vi "newGUI.vi"() -> ()   [LabVIEW 2021]
uses:
  UI Data.ctl
  Data.ctl
  <vilib>/Instr/_visa.llb/VISA Flush IO Buffer Mask.ctl
  f08f8e5a-3cc6-4510-ab96-cacb044e89f4.vi
  816ef2ce-0aac-4e16-9f0f-254035a33ee7.vi
  7bf0c881-b533-49c5-b976-3a179d9b9c35.vi
  5e66b44c-e304-46e7-babf-65c984714624.vi
  a6c2df6f-6ad4-4eb4-a9bc-2f05b466e969.vi
  d2f15d41-d429-4762-bc4d-8d0cbb89ed83.vi
  535851f3-05c5-415e-8a07-50860e4f08cf.vi
  3643a199-7bcb-4f24-a83d-5ca93d957abf.vi
  187f9bc3-0ed3-4701-b56c-3ff7ee860393.vi
  eb7b7dfd-645e-46e6-868f-ba0f7f713db4.vi
  <vilib>/Instr/_visa.llb/VISA Configure Serial Port (Instr).vi
  styles/colors.vi
  <vilib>/ULx/ULx_LV.dll
  <vilib>/ULx/Write.llb/ULx Write (Digital Bool 1Line 1Point).vi
  <vilib>/NI/Progress Bar/Progress Bar.lvlib
  <vilib>/zip/NI_Unzip.lvlib
  <vilib>/ULx/Create Channel.llb/ULx Create Channel (DO-Digital Output).vi
panel:
  in  "Stop button":bool
  in  "Run button":bool
  in  "Settings button":bool
  out "Console":string
  in  "Serial communication\n settings":T1={"COM"="", "baud rate"=115200, "data bits"=8, "parity"=enum."None", "stop bits"=10, "flow control"=enum."None", "delay"=50, "I/O channel"=""} {"stop bits" items=["1.0"=10, "1.5"=15, "2.0"=20]; "baud rate" max=921600; "data bits" max=16}
  in  "Paths":bool
  in  "Save button":bool
  in  "Path: 4.9.12.XXXX":path=path "C:/Users/ken_X/Documents/LabVIEW projects/Project-A/outset-medical/4.9.12.6034"
  in  "Path: Android OS":path=path "C:/Users/ken_X/Documents/LabVIEW projects/Project-A/outset-medical/Android OS"
  # "Serial communication\n settings"
  # "I/O Channel"
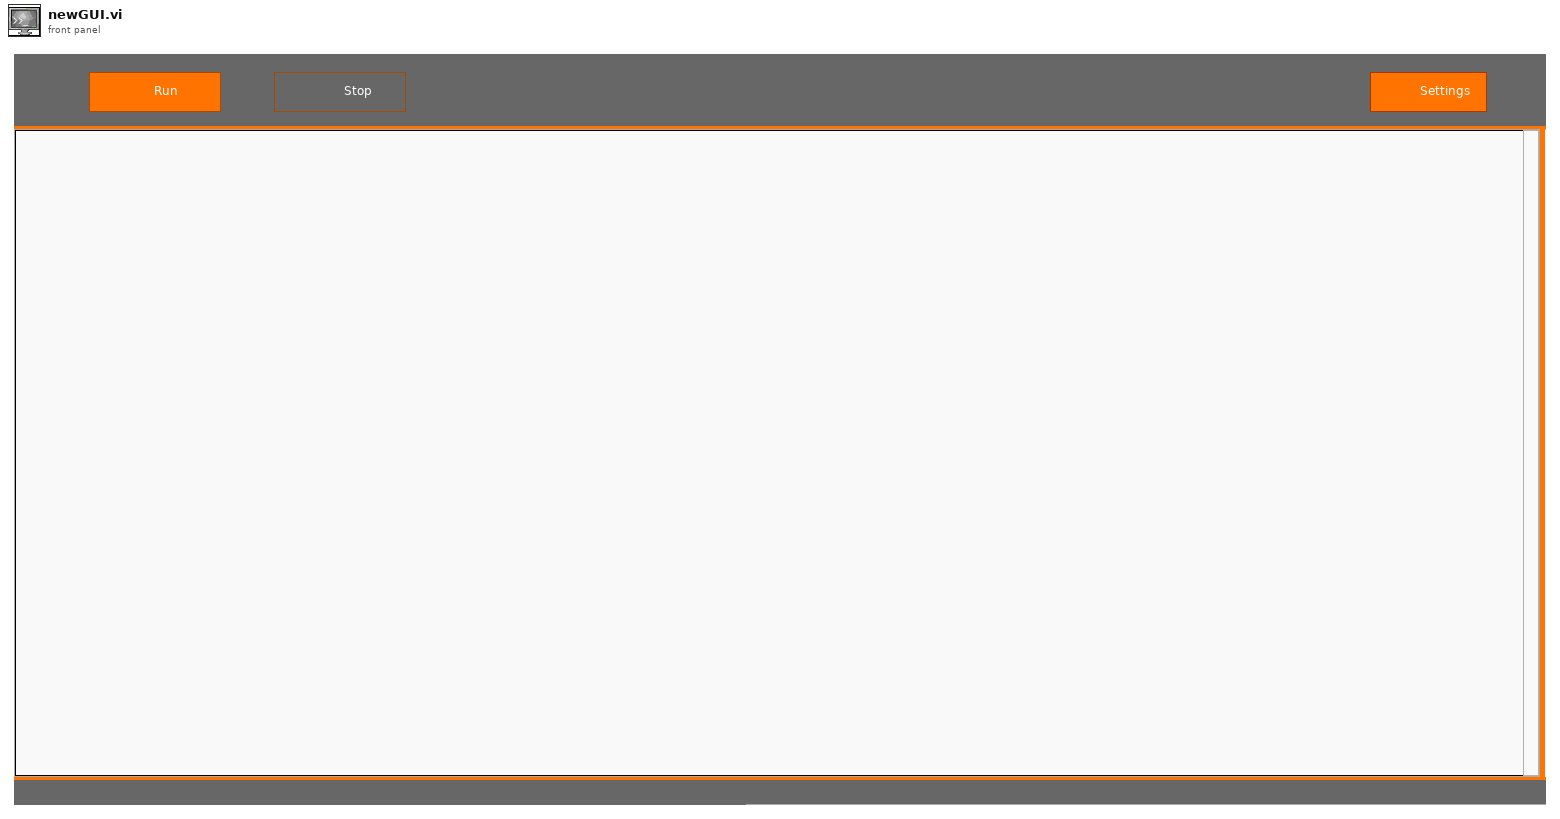
[diagram p1: front panel]
types:
  T1 = cluster{"COM":refnum<visa-resource-name>, "baud rate":u32, "data bits":u8, "parity":enum16{"None", "Odd", "Even", "Mark", "Space"}, "stop bits":u16, "flow control":enum16{"None", "XON/XOFF", "RTS/CTS", "DTR/DSR"}, "delay":u16, "I/O channel":refnum<k21>}
  T2 = typedef "Data.ctl" = cluster{"Console":refnum<vi>, "COM":refnum<visa-resource-name>, "Delay":u32, "IO task":refnum<k24>, "Python session":refnum<k35>, "Script path":path, "Media Url":string, "Media version":i32, "Attempts left":i32, "Version path":path, "Android path":path, "Python 2.7":path, "My temp":path}
  T3 = enum8{"Enabled", "Disabled", "Disabled and Grayed Out"}
  T4 = typedef "UI Data.ctl" = cluster{"settings splitter":refnum<vi>, "footer splitter":refnum<vi>, "Serial communication\n settings":refnum<vi>, "Path: Android OS":refnum<vi>, "Path: 4.9.12.XXXX":refnum<vi>}
  T5 = cluster{"primary color":u32, "secondary color":u32, "accent color":u32, "background color":u32, "accent s color":u32}
  T6 = cluster{"accent s color":u32, "accent s color":u32}
  T7 = cluster{"accent s color":u32, "accent color":u32}
  T8 = cluster{"primary color":u32, "primary color":u32}
  T9 = enum16{"open", "replace", "create", "open or create", "replace or create", "replace or create with confirmation"}
  T10 = cluster{"Android":path, "Version":path, "Labview Script":path, "Python 2.7":path, "My temp":path}
  T11 = typedef "VISA Flush IO Buffer Mask.ctl" = u16
  T12 = cluster{"secondary color":u32, "secondary color":u32}
  T13 = cluster{"Value":path, "Value":path, path, path, path}
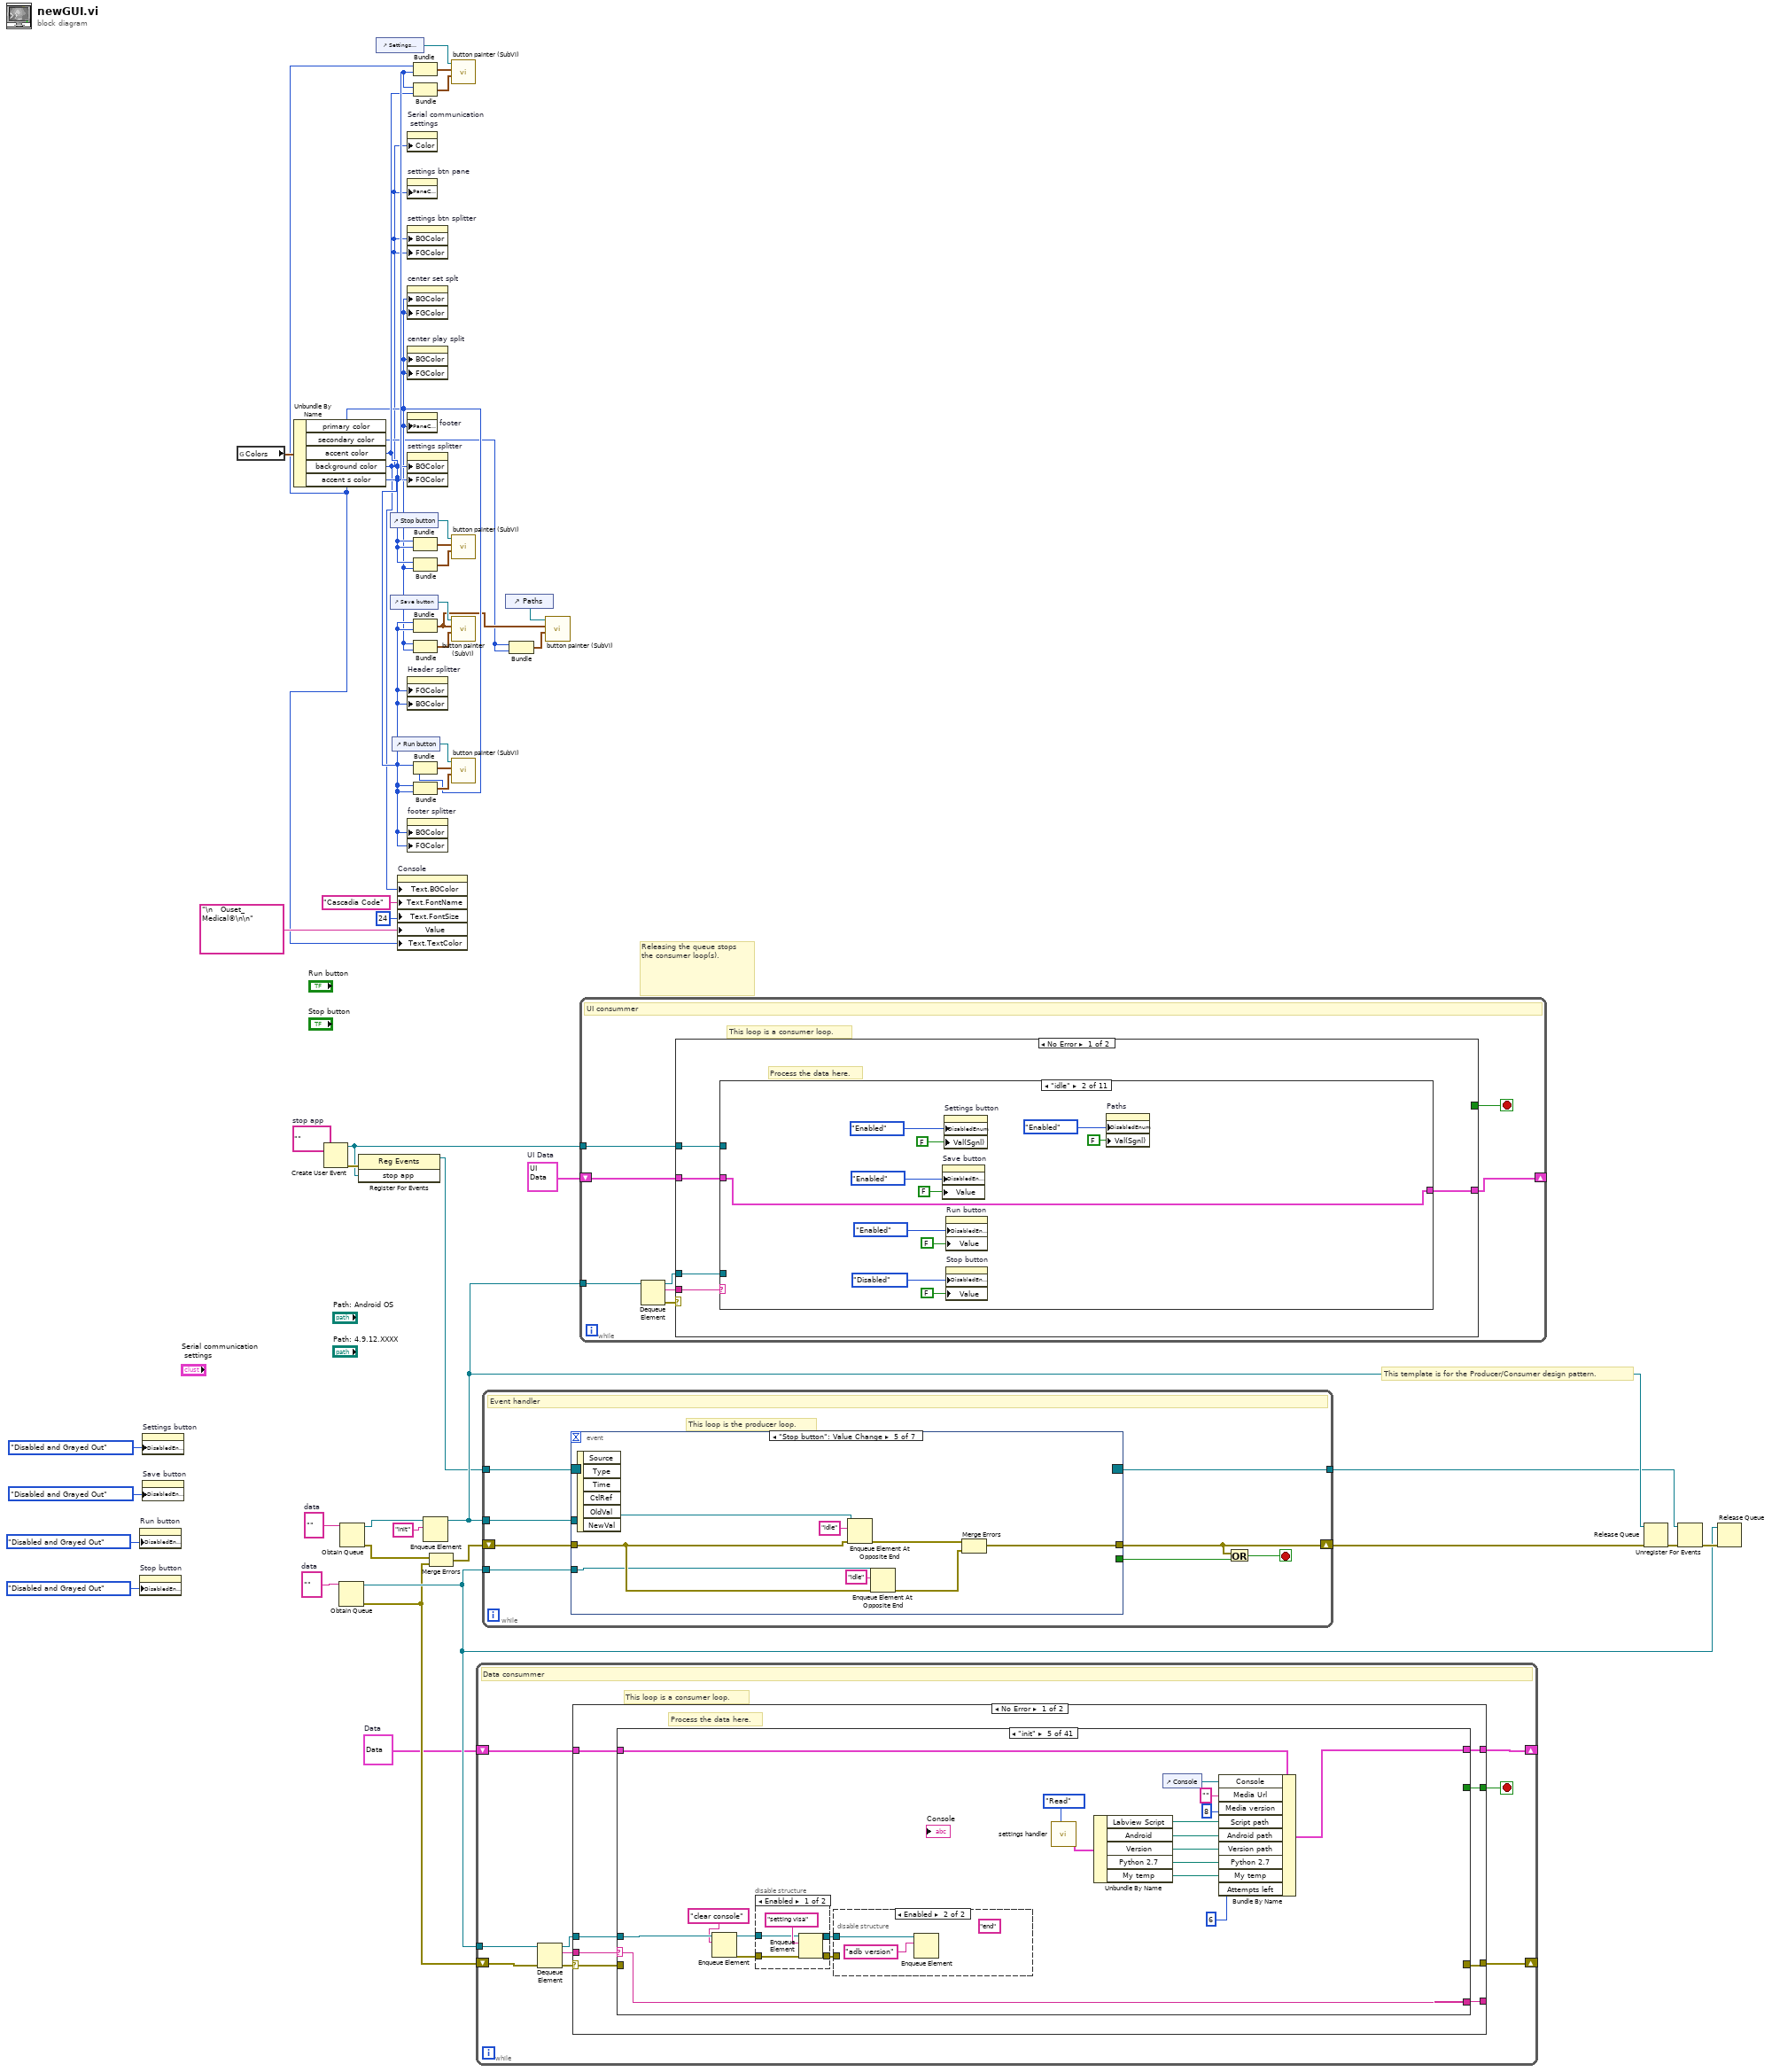
[diagram p0: block diagram]
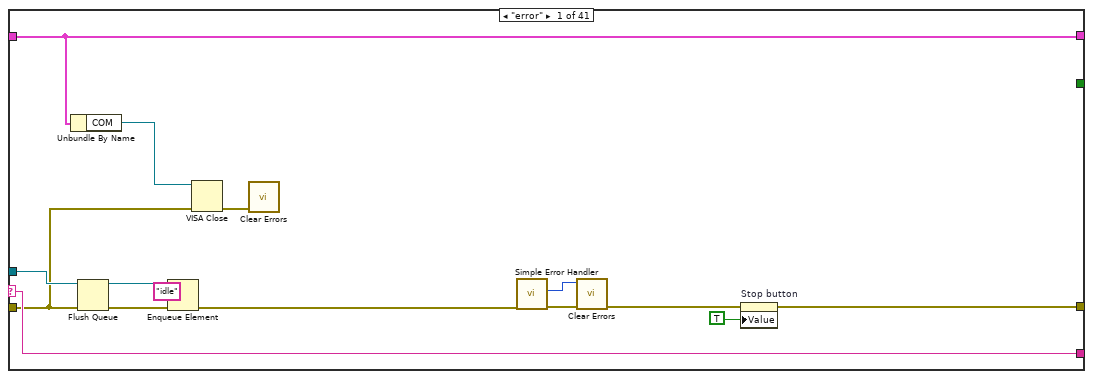
[diagram p2: hidden frame]
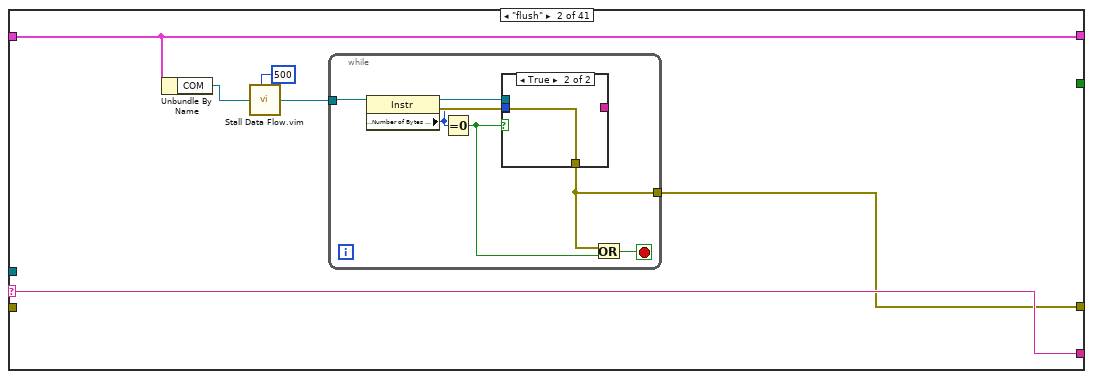
[diagram p3: hidden frame]
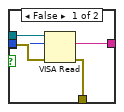
[diagram p4: hidden frame]
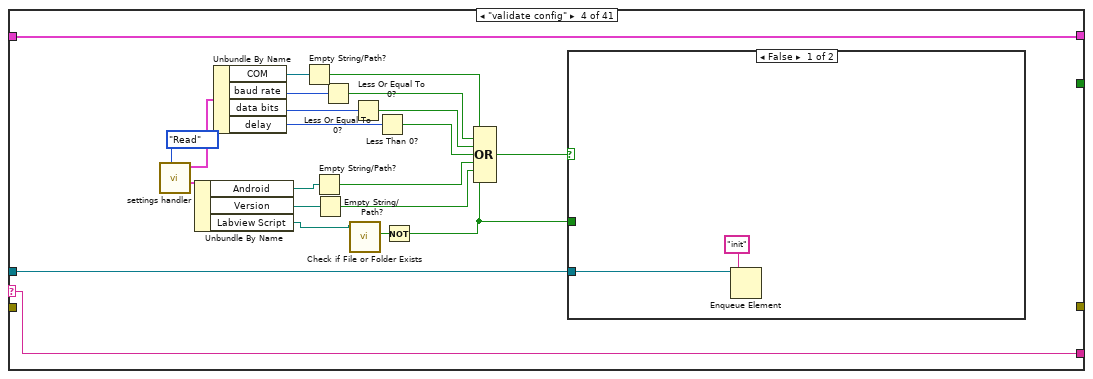
[diagram p6: hidden frame]
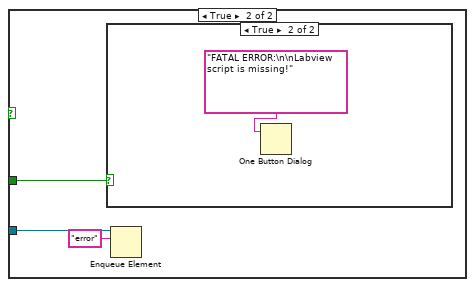
[diagram p7: hidden frame]
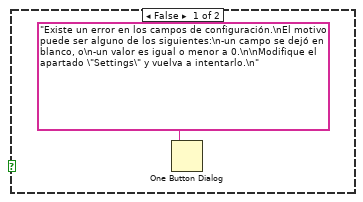
[diagram p8: hidden frame]
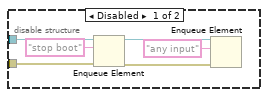
[diagram p10: hidden frame]
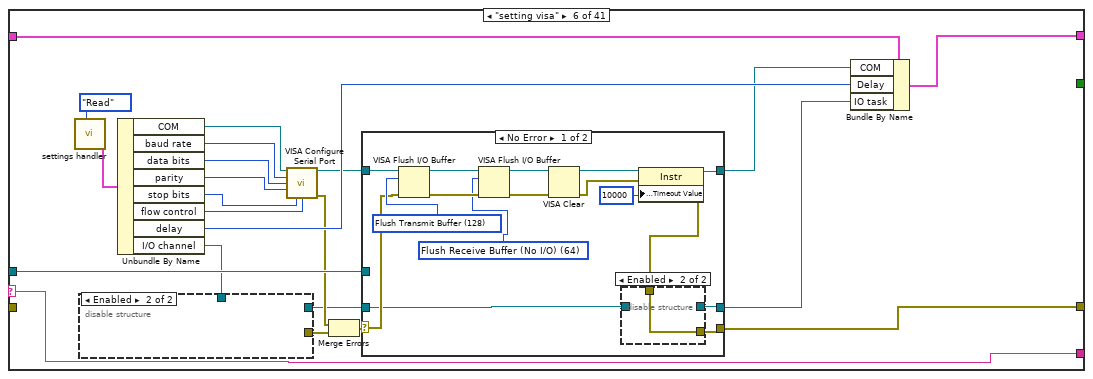
[diagram p11: hidden frame]
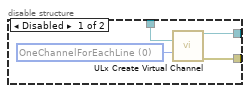
[diagram p12: hidden frame]
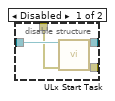
[diagram p13: hidden frame]
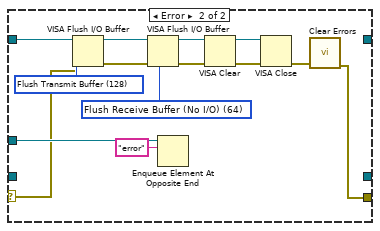
[diagram p14: hidden frame]
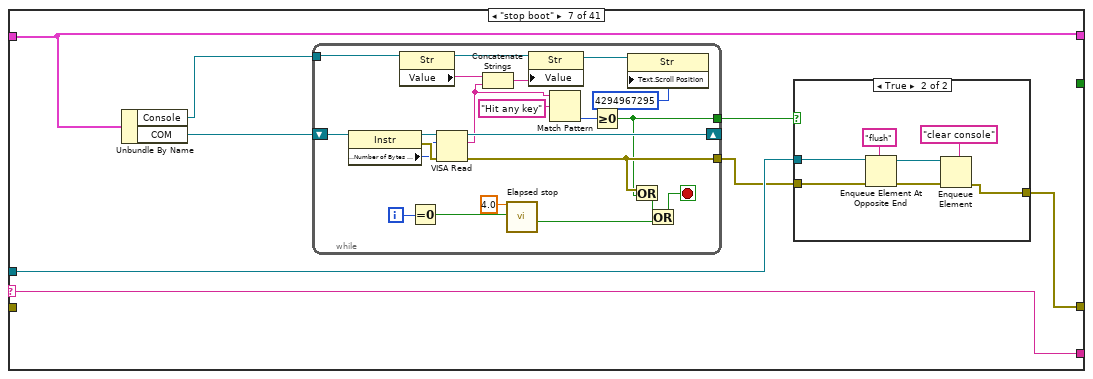
[diagram p15: hidden frame]
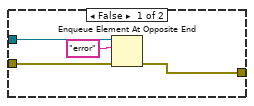
[diagram p16: hidden frame]
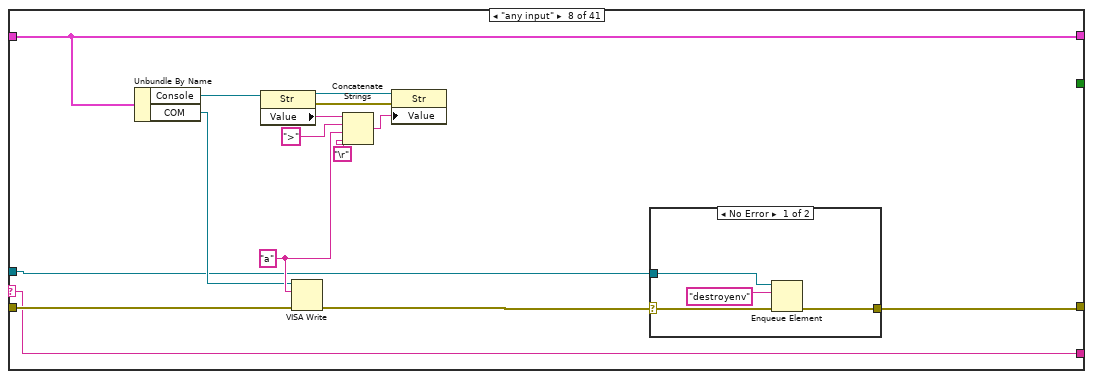
[diagram p17: hidden frame]
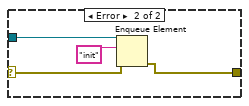
[diagram p18: hidden frame]
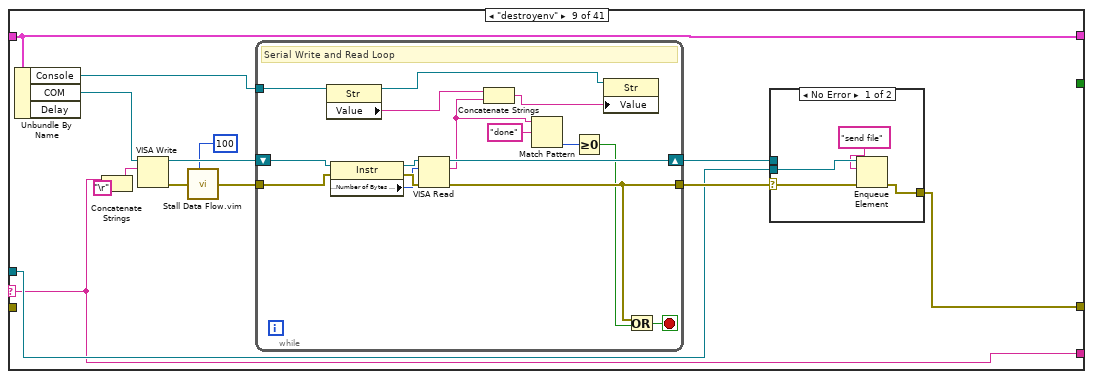
[diagram p19: hidden frame]
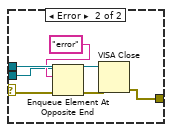
[diagram p20: hidden frame]
diagram:
  w2 = T2 {"Console"=refnum, "COM"="", "Delay"=50, "IO task"=refnum, "Python session"=refnum, "Script path"=path "C:/Users/ken_X/Documents/LabVIEW projects/Project-A/Update_Media_bi.py", "Media Url"="", "Media version"=0, "Attempts left"=3, "Version path"=path "C:/Users/ken_X/Documents/LabVIEW projects/Project-A/Update_Media_bi.py", "Android path"=path "C:/Users/ken_X/Documents/LabVIEW projects/Project-A/Update_Media_bi.py", "Python 2.7"=path "C:/Users/ken_X/Documents/LabVIEW projects/Project-A/Update_Media_bi.py", "My temp"=path "C:/Users/ken_X/Documents/LabVIEW projects/Project-A/Update_Media_bi.py"}  # Data
  w22 = ""  # data
  w37 = ""  # stop app
  w41 = T4 {"settings splitter"=refnum, "footer splitter"=refnum, "Serial communication\n settings"=refnum, "Path: Android OS"=refnum, "Path: 4.9.12.XXXX"=refnum}  # UI Data
  w38 = ""  # data
  # "Releasing the queue stops the consumer loop(s)."
  # "This template is for the Producer/Consumer design pattern."
  n1 = property on="Run button" class="Bool (strict)"("DisabledEnum"=T3."Disabled and Grayed Out" ("Disabled")) -> ()  [unwired: 2 in, 2 out]
  n2 = property on="Stop button" class="Bool (strict)"("DisabledEnum"=T3."Disabled and Grayed Out" ("Disabled")) -> ()  [unwired: 2 in, 2 out]
  n3 = property on="Settings button" class="Bool (strict)"("DisabledEnum"=T3."Disabled and Grayed Out" ("Disabled")) -> ()  [unwired: 2 in, 2 out]
  n4 = property on="Save button" class="Bool (strict)"("DisabledEnum"=T3."Disabled and Grayed Out" ("Disabled")) -> ()  [unwired: 2 in, 2 out]
  n5 = global read "colors.vi" "Colors"() -> (w46:T5)
  n6 = Unbundle By Name(w46) -> ("primary color"=w9:u32, "secondary color"=w5:u32, "accent color"=w10:u32, "background color"=w3:u32, "accent s color"=w11:u32)
  n7 = Create User Event(user event datatype=w37) -> (user event=w35:refnum<user-event>, error out=w36:errorcluster)  [unwired: 1 in]
  n8 = Obtain Queue(element data type=w22) -> (queue out=w18:refnum<queue>, error out=w17:errorcluster)  [unwired: 4 in, 1 out]
  n9 = Obtain Queue(element data type=w38) -> (queue out=w44:refnum<queue>, error out=w21:errorcluster)  [unwired: 4 in, 1 out]
  n10 = register-events(error in=w36, w35) -> (reference out=w1:refnum<event-registration>)  [unwired: 1 in, 1 out]
  n11 = control-ref of="Settings button"() -> (w27:refnum<vi>)
  n12 = control-ref of="Stop button"() -> (w25:refnum<vi>)
  n13 = control-ref of="Save button"() -> (w26:refnum<vi>)
  n14 = control-ref of="Run button"() -> (w32:refnum<vi>)
  n15 = property on="Console" class="Str"("Text.BGColor"=w3, "Text.FontName"="Cascadia Code" ("Text.Font:Name"), "Text.FontSize"=u32 24 ("Text.Font:Size"), "Value"="\n   Ouset_Medical®\n\n" ("Console"), "Text.TextColor"=w11) -> ()  [unwired: 2 in, 2 out]
  n16 = property on="Serial communication\n settings" class="Clust (strict)"("Color"=w3) -> ()  [unwired: 2 in, 2 out]
  n17 = property on="settings btn pane" class="Pane"("PaneColor"=w3) -> ()  [unwired: 2 in, 2 out]
  n18 = property on="settings btn splitter" class="Splitter"("BGColor"=w3, "FGColor"=w3) -> ()  [unwired: 2 in, 2 out]
  n19 = property on="center set splt" class="Splitter"("BGColor"=w9, "FGColor"=w9) -> ()  [unwired: 2 in, 2 out]
  n20 = property on="center play split" class="Splitter"("BGColor"=w9, "FGColor"=w9) -> ()  [unwired: 2 in, 2 out]
  n21 = property on="footer" class="Pane"("PaneColor"=w9) -> ()  [unwired: 2 in, 2 out]
  n22 = property on="settings splitter" class="Splitter"("BGColor"=w10, "FGColor"=w10) -> ()  [unwired: 2 in, 2 out]
  n23 = property on="Header splitter" class="Splitter"("FGColor"=w10, "BGColor"=w10) -> ()  [unwired: 2 in, 2 out]
  n24 = property on="footer splitter" class="Splitter"("BGColor"=w10, "FGColor"=w10) -> ()  [unwired: 2 in, 2 out]
  n25 = Bundle("accent s color"=w11, "accent s color"=w11) -> (w29:T6)  [unwired: 1 in]
  n26 = Bundle("accent s color"=w11, "accent color"=w10) -> (w28:T7)  [unwired: 1 in]
  n27 = Bundle("accent color"=w10, "accent color"=w10) -> (w23:cluster{"accent color":u32, "accent color":u32})  [unwired: 1 in]
  n28 = Bundle("accent color"=w10, "primary color"=w9) -> (w24:cluster{"accent color":u32, "primary color":u32})  [unwired: 1 in]
  n29 = Bundle("accent color"=w10, "accent color"=w10) -> (w7:cluster{"accent color":u32, "accent color":u32})  [unwired: 1 in]
  n30 = Bundle("primary color"=w9, "primary color"=w9) -> (w6:T8)  [unwired: 1 in]
  n31 = Bundle("accent color"=w10, "primary color"=w9) -> (w30:cluster{"accent color":u32, "primary color":u32})  [unwired: 1 in]
  n32 = Bundle("accent color"=w10, "accent color"=w10) -> (w31:cluster{"accent color":u32, "accent color":u32})  [unwired: 1 in]
  n33 = Enqueue Element(queue=w44, element="init") -> (queue out=w43:refnum<queue>)  [unwired: 2 in, 2 out]
  n34 = Merge Errors(w21, w17) -> (w20:errorcluster)
  n35 = call "button painter (SubVI).vi"("Off state"=w28, "On state"=w29, "Button ref in"=w27) -> ()  [unwired: 9 in]
  n36 = call "button painter (SubVI).vi"("Off state"=w24, "On state"=w23, "Button ref in"=w25) -> ()  [unwired: 9 in]
  n37 = call "button painter (SubVI).vi"("Off state"=w6, "On state"=w7, "Button ref in"=w26) -> ()  [unwired: 9 in]
  n38 = call "button painter (SubVI).vi"("Off state"=w31, "On state"=w30, "Button ref in"=w32) -> ()  [unwired: 9 in]
  n39 = while {
    tunnel: w18 -> [w55]
    shift-right: [w49] -> _
    shift-left: w2 -> [w50]
    shift-right: [w47] -> _
    shift-left: w17 -> [w51]
    stop <- w48 stop-if-true
    # "This loop is a consumer loop."
    # "Data consummer"
    n40 = Dequeue Element(queue=w55, error in (no error)=w51) -> (queue out=w52:refnum<queue>, element=w53:string, error out=w54:errorcluster)  [unwired: 1 in, 1 out]
    n41 = case shown="No Error" w54 {
      selector: w54 -> [w58 w1281]
      tunnel: w53 -> [w63 _]
      tunnel: w52 -> [w62 w1285]
      tunnel: w50 -> [w61 w1284]
      tunnel: [w60 w1284] -> w49
      tunnel: [w59 "ERROR"] -> _
      tunnel: [w57 w1277] -> w47
      tunnel: [w56 _] -> w48
      frame No Error {
        # "Process the data here."
        n42 = case shown="\"init\"" w63 {
          selector: w63 -> [w75 w83 w98 w103 w144 w166 w231 w266 w294 w350 w370 w398 w456 w486 w490 w520 w539 w583 w630 w662 w690 w716 w746 w795 w817 w862 w881 w901 w933 w977 w1012 w1038 w1060 w1092 w1124 w1150 w1191 w1222 w1236 w1240 w1256]
          tunnel: w62 -> [w77 _ _ w104 w148 w174 w232 w267 w298 w352 w374 w401 w447 _ _ w510 w546 w584 w633 w664 w692 w717 w748 w797 w819 w864 _ w894 w926 w971 w1014 w1035 w1063 w1095 w1127 w1152 w1193 w1224 _ _ w1252]
          tunnel: w61 -> [w78 w84 w99 w121 w147 w179 w229 w280 w297 w351 w371 w395 w455 w489 w492 w494 w555 w581 w620 w669 w701 w722 w756 w798 w828 w869 w877 w899 w925 w968 w1023 w1040 w1051 w1083 w1115 w1156 w1183 w1215 w1235 w1241 w1251]
          tunnel: [w78 w84 w99 w121 w145 w178 w229 w280 w297 w351 w371 w395 w455 w488 w492 w494 w555 w581 w619 w669 w701 w722 w756 w798 w828 w869 w877 w892 w925 w967 w1023 w1040 w1051 w1083 w1115 w1156 w1183 w1215 w1235 w1241 w1251] -> w60
          tunnel: [w75 w83 w98 w103 w144 w166 w231 w266 w294 w350 w370 w398 w456 w486 w490 w520 w539 w583 w630 w662 w690 w716 w746 w795 w817 w862 w881 w901 w933 w977 w1012 w1038 w1060 w1092 w1124 w1150 w1191 w1222 w1236 w1240 w1256] -> w59
          tunnel: w58 -> [w71 _ _ _ _ _ _ w271 _ _ _ _ _ _ _ w508 w544 _ w627 _ w687 w714 w739 _ _ _ w879 w897 w929 _ w1013 w1037 _ _ _ w1153 _ _ _ _ _]
          tunnel: [w65 w79 _ _ _ w164 w226 w268 w289 w338 w369 w396 w446 w485 _ w506 w543 w578 w628 w663 w688 w715 w740 w785 w815 w850 w878 w893 w927 w972 w1011 w1036 w1058 w1090 w1122 w1154 w1189 w1220 _ _ w1253] -> w57
          tunnel: [_ _ _ _ _ _ _ _ _ _ _ _ _ _ _ _ _ _ _ _ _ _ _ _ _ _ _ _ _ _ _ _ _ _ _ _ _ _ _ TRUE _] -> w56
          frame "error" {
            n43 = Unbundle By Name(w78) -> ("COM"=w72:refnum<visa-resource-name>)
            n44 = Flush Queue(queue=w77, error in (no error)=w71) -> (queue out=w74:refnum<queue>, error out=w73:errorcluster)  [unwired: 1 out]
            n45 = Enqueue Element(queue=w74, element="idle", error in (no error)=w73) -> (error out=w66:errorcluster)  [unwired: 1 in, 2 out]
            n46 = VISA Close(VISA resource name=w72, error in (no error)=w71) -> (error out=w64:errorcluster)
            n47 = call <vilib>:"Clear Errors.vi"("error in (no error)"=w64) -> ()  [unwired: 5 in, 2 out]
            n48 = call <vilib>:"Simple Error Handler.vi"("error in (no error)"=w66) -> ("code out"=w69:i32, "error out"=w68:errorcluster)  [unwired: 4 in, 3 out]
            n49 = call <vilib>:"Clear Errors.vi"("error in (no error)"=w68, "specific error code to clear (0: all)"=w69) -> ("error out"=w67:errorcluster)  [unwired: 4 in, 1 out]
            n50 = property on="Stop button" class="Bool (strict)"(error in=w67, "Value"=TRUE ("Value (Signaling)")) -> (error out=w65:errorcluster)  [unwired: 1 in, 1 out]
          }
          frame "flush" {
            n51 = Unbundle By Name(w84) -> ("COM"=w82:refnum<visa-resource-name>)
            n52 = call "Stall Data Flow.vim"("value in"=w82, "milliseconds to wait"=u32 500) -> ("value out"=w81:refnum<visa-resource-name>)  [unwired: 1 out]
            n53 = while {
              tunnel: w81 -> [w91]
              tunnel: [w85] -> w79
              stop <- w89 stop-if-true
              n54 = property class="Instr"(reference=w91) -> (reference out=w90:refnum<visa-resource-name>, error out=w88:errorcluster, "Serial Settings:Number of Bytes at Serial Port"=w86:u32)  [unwired: 1 in]
              n55 = Equal To 0?(x=w86) -> (x = 0?=w87:bool)
              n56 = case shown="True" w87 {
                tunnel: w90 -> [w96 _]
                tunnel: w88 -> [w95 w97]
                tunnel: [w94 w97] -> w85
                tunnel: w86 -> [w93 _]
                tunnel: [w92 _] -> _
                frame False {
                  n57 = VISA Read(VISA resource name=w96, byte count=w93, error in (no error)=w95) -> (read buffer=w92:string, error out=w94:errorcluster)  [unwired: 2 out]
                }
                frame True {
                }
              }
              n58 = Or(x=w85, y=w87) -> (x .or. y?=w89:bool)
            }
          }
          frame "idle", Default {
          }
          frame "validate config" {
            n59 = call "settings handler.vi"("Operation"=enum16{"Open", "Write", "Read", "Close"}."Read") -> ("Paths read"=w119:T10, "Read"=w114:T1)  [unwired: 8 in, 1 out]
            n60 = Unbundle By Name(w119) -> ("Android"=w117:path, "Version"=w118:path, "Labview Script"=w102:path)
            n61 = Unbundle By Name(w114) -> ("COM"=w113:refnum<visa-resource-name>, "baud rate"=w112:u32, "data bits"=w111:u8, "delay"=w110:u16)
            n62 = Empty String/Path?(string/path=w113) -> (empty?=w106:bool)
            n63 = Empty String/Path?(string/path=w117) -> (empty?=w115:bool)
            n64 = Empty String/Path?(string/path=w118) -> (empty?=w116:bool)
            n65 = Less Or Equal To 0?(x=w112) -> (x <= 0?=w107:bool)
            n66 = call <vilib>:"Check if File or Folder Exists.vi"("path"=w102) -> ("file or folder exists?"=w101:bool)  [unwired: 8 in, 2 out]
            n67 = Less Or Equal To 0?(x=w111) -> (x <= 0?=w108:bool)
            n68 = Less Than 0?(x=w110) -> (x < 0?=w109:bool)
            n69 = Not(x=w101) -> (.not. x?=w100:bool)
            n70 = Compound Arithmetic op=OR(w106, w107, w108, w109, w115, w116, w100) -> (w105:bool)
            n71 = case shown="False" w105 {
              tunnel: w104 -> [w123 w126]
              tunnel: w100 -> [_ w124]
              frame False {
                n72 = Enqueue Element(queue=w123, element="init") -> ()  [unwired: 2 in, 3 out]
              }
              frame True {
                n73 = case shown="True" w124 {
                  frame False {
                    n74 = One Button Dialog(message="Existe un error en los campos de configuración.\nEl motivo puede ser alguno de los siguientes:\n-un campo se dejó en blanco, o\n-un valor es igual o menor a 0.\n\nModifique el apartado \"Settings\" y vuelva a intentarlo.\n") -> ()  [unwired: 1 in, 1 out]
                  }
                  frame True {
                    n75 = One Button Dialog(message="FATAL ERROR:\n\nLabview script is missing!") -> ()  [unwired: 1 in, 1 out]
                  }
                }
                n76 = Enqueue Element(queue=w126, element="error") -> ()  [unwired: 2 in, 3 out]
              }
            }
          }
          frame "init" {
            n77 = Enqueue Element(queue=w148, element="clear console") -> (queue out=w143:refnum<queue>, error out=w134:errorcluster)  [unwired: 2 in, 1 out]
            n78 = disable-structure shown="Enabled" {
              disable-tunnel: w143 -> [w152 w155]
              disable-tunnel: [w151 w155] -> w141
              disable-tunnel: [w150 w154] -> w135
              disable-tunnel: w134 -> [w149 w154]
              frame Enabled {
                n79 = Enqueue Element(queue=w152, element="setting visa", error in (no error)=w149) -> (queue out=w151:refnum<queue>, error out=w150:errorcluster)  [unwired: 1 in, 1 out]
              }
              frame Disabled {
              }
            }
            n80 = disable-structure shown="Enabled" {
              disable-tunnel: w141 -> [w161 w163]
              disable-tunnel: w135 -> [w157 _]
              frame Disabled {
                n81 = Enqueue Element(queue=w161, element="stop boot", error in (no error)=w157) -> (queue out=w159:refnum<queue>, error out=w158:errorcluster)  [unwired: 1 in, 1 out]
                n82 = Enqueue Element(queue=w159, element="any input", error in (no error)=w158) -> ()  [unwired: 1 in, 3 out]
              }
              frame Enabled {
                (unwired) "end" ("element")
                n83 = Enqueue Element(queue=w163, element="adb version") -> ()  [unwired: 2 in, 3 out]
              }
            }
            n84 = call "settings handler.vi"("Operation"=enum16{"Open", "Write", "Read", "Close"}."Read") -> ("Paths read"=w137:T10)  [unwired: 8 in, 2 out]
            n85 = Unbundle By Name(w137) -> ("Labview Script"=w136:path, "Android"=w132:path, "Version"=w131:path, "Python 2.7"=w130:path, "My temp"=w129:path)
            n86 = control-ref of="Console"() -> (w146:refnum<vi>)
            n87 = Bundle By Name(cluster=w147, "Console"=w146, "Media Url"="", "Media version"=8, "Script path"=w136, "Android path"=w132, "Version path"=w131, "Python 2.7"=w130, "My temp"=w129, "Attempts left"=6) -> (w145:T2)
          }
          frame "setting visa" {
            n88 = call "settings handler.vi"("Operation"=enum16{"Open", "Write", "Read", "Close"}."Read") -> ("Read"=w184:T1)  [unwired: 8 in, 2 out]
            n89 = Unbundle By Name(w184) -> ("COM"=w183:refnum<visa-resource-name>, "baud rate"=w182:u32, "data bits"=w181:u8, "parity"=w180:enum16{"None", "Odd", "Even", "Mark", "Space"}, "stop bits"=w176:u16, "flow control"=w177:enum16{"None", "XON/XOFF", "RTS/CTS", "DTR/DSR"}, "delay"=w175:u16, "I/O channel"=w167:refnum<k21>)
            n90 = disable-structure shown="Enabled" {
              disable-tunnel: [w189 _] -> w170
              disable-tunnel: [w188 _] -> w169
              disable-tunnel: w167 -> [w187 _]
              frame Disabled {
                w186 = 0 items=["OneChannelForEachLine", "OneChannelForAllLines"] ("line grouping")
                n91 = call-poly <vilib>:"ULx Create Virtual Channel.vi"("lines"=w187, "line grouping"=w186) -> ("task out"=w188:refnum<k24>, "error out"=w189:errorcluster)  [unwired: 12 in]
              }
              frame Enabled {
              }
            }
            n92 = call-poly "VISA Configure Serial Port"("VISA resource name"=w183, "baud rate (9600)"=w182, "data bits (8)"=w181, "parity (0:none)"=w180, "stop bits (10: 1 bit)"=w176, "flow control (0:none)"=w177) -> ("VISA resource name out"=w173:refnum<visa-resource-name>, "error out"=w171:errorcluster)  [unwired: 4 in, 4 out]
            n93 = Merge Errors(w171, w170) -> (w172:errorcluster)
            n94 = case shown="No Error" w172 {
              selector: w172 -> [w201 w216]
              tunnel: w174 -> [_ w224]
              tunnel: w173 -> [w203 w221]
              tunnel: [w197 w215] -> w164
              tunnel: [w199 _] -> w168
              tunnel: w169 -> [w200 _]
              tunnel: [w204 _] -> w165
              frame No Error {
                w194 = T11 64 items=["Flush Receive Buffer"=16, "Write Transmit Buffer to Device"=32, "Flush Receive Buffer (No I/O)"=64, "Flush Transmit Buffer"=128] ("Mask")
                w202 = T11 128 items=["Flush Receive Buffer"=16, "Write Transmit Buffer to Device"=32, "Flush Receive Buffer (No I/O)"=64, "Flush Transmit Buffer"=128] ("Mask")
                n95 = VISA Flush I/O Buffer(VISA resource name=w203, mask (16)=w202, error in (no error)=w201) -> (VISA resource name out=w196:refnum<visa-resource-name>, error out=w195:errorcluster)
                n96 = VISA Flush I/O Buffer(VISA resource name=w196, mask (16)=w194, error in (no error)=w195) -> (VISA resource name out=w193:refnum<visa-resource-name>, error out=w192:errorcluster)
                n97 = VISA Clear(VISA resource name=w193, error in (no error)=w192) -> (VISA resource name out=w191:refnum<visa-resource-name>, error out=w190:errorcluster)
                n98 = property class="Instr"(reference=w191, error in=w190, "General Settings:Timeout Value"=u32 10000) -> (reference out=w204:refnum<visa-resource-name>, error out=w198:errorcluster)
                n99 = disable-structure shown="Enabled" {
                  disable-tunnel: w200 -> [w209 _]
                  disable-tunnel: [w208 _] -> w199
                  disable-tunnel: w198 -> [w207 w210]
                  disable-tunnel: [w206 w210] -> w197
                  frame Disabled {
                    n100 = call <vilib>:"ULx Start Task.vi"("task in"=w209, "error in"=w207) -> ("task out"=w208:refnum<k24>, "error out"=w206:errorcluster)  [unwired: 12 in]
                  }
                  frame Enabled {
                  }
                }
              }
              frame Error {
                w218 = T11 64 items=["Flush Receive Buffer"=16, "Write Transmit Buffer to Device"=32, "Flush Receive Buffer (No I/O)"=64, "Flush Transmit Buffer"=128] ("Mask")
                w219 = T11 128 items=["Flush Receive Buffer"=16, "Write Transmit Buffer to Device"=32, "Flush Receive Buffer (No I/O)"=64, "Flush Transmit Buffer"=128] ("Mask")
                n101 = VISA Flush I/O Buffer(VISA resource name=w221, mask (16)=w219, error in (no error)=w216) -> (VISA resource name out=w220:refnum<visa-resource-name>, error out=w217:errorcluster)
                n102 = VISA Flush I/O Buffer(VISA resource name=w220, mask (16)=w218, error in (no error)=w217) -> (VISA resource name out=w214:refnum<visa-resource-name>, error out=w213:errorcluster)
                n103 = Enqueue Element At Opposite End(queue=w224, element="error") -> ()  [unwired: 2 in, 3 out]
                n104 = VISA Clear(VISA resource name=w214, error in (no error)=w213) -> (VISA resource name out=w212:refnum<visa-resource-name>, error out=w211:errorcluster)
                n105 = VISA Close(VISA resource name=w212, error in (no error)=w211) -> (error out=w222:errorcluster)
                n106 = call <vilib>:"Clear Errors.vi"("error in (no error)"=w222) -> ("error out"=w215:errorcluster)  [unwired: 5 in, 1 out]
              }
            }
            n107 = Bundle By Name(cluster=w179, "COM"=w165, "Delay"=w175, "IO task"=w168) -> (w178:T2)
          }
          frame "stop boot" {
            n108 = Unbundle By Name(w229) -> ("Console"=w225:refnum<vi>, "COM"=w227:refnum<visa-resource-name>)
            n109 = while {
              shift-right: [w254] -> _
              shift-left: w227 -> [w251]
              tunnel: [w253] -> w228
              tunnel: [w247] -> w230
              tunnel: w225 -> [w233]
              i -> [w242]
              stop <- w245 stop-if-true
              # "Serial Write and Read Loop"
              n110 = property class="Instr"(reference=w251) -> (reference out=w250:refnum<visa-resource-name>, error out=w249:errorcluster, "Serial Settings:Number of Bytes at Serial Port"=w248:u32)  [unwired: 1 in]
              n111 = property class="Str"(reference=w233) -> (reference out=w240:refnum<vi>, "Value"=w237:string)  [unwired: 1 in, 1 out]
              n112 = Equal To 0?(x=w242) -> (x = 0?=w241:bool)
              n113 = VISA Read(VISA resource name=w250, byte count=w248, error in (no error)=w249) -> (VISA resource name out=w254:refnum<visa-resource-name>, read buffer=w236:string, error out=w253:errorcluster)  [unwired: 1 out]
              n114 = Concatenate Strings(w237, w236) -> (w238:string)
              n115 = call "Elapsed stop"("Time Target (s)"=4.0, "Reset"=w241) -> ("Time has Elapsed"=w244:bool)  [unwired: 10 in, 7 out]
              n116 = property class="Str"(reference=w240, "Value"=w238) -> (reference out=w235:refnum<vi>)  [unwired: 1 in, 1 out]
              n117 = Match Pattern(string=w236, regular expression="Hit any key") -> (offset past match=w252:i32)  [unwired: 1 in, 3 out]
              n118 = Greater Or Equal To 0?(x=w252) -> (x >= 0?=w247:bool)
              n119 = property class="Str"(reference=w235, "Text.Scroll Position"=u32 4294967295) -> ()  [unwired: 1 in, 2 out]
              n120 = Or(x=w253, y=w247) -> (x .or. y?=w246:bool)
              n121 = Or(x=w246, y=w244) -> (x .or. y?=w245:bool)
            }
            n122 = case shown="True" w230 {
              tunnel: w232 -> [w258 w259]
              tunnel: w228 -> [w256 w263]
              tunnel: [w255 w261] -> w226
              frame False {
                n123 = Enqueue Element At Opposite End(queue=w258, element="error", error in (no error)=w256) -> (error out=w255:errorcluster)  [unwired: 1 in, 2 out]
              }
              frame True {
                n124 = Enqueue Element At Opposite End(queue=w259, element="flush", error in (no error)=w263) -> (queue out=w260:refnum<queue>, error out=w262:errorcluster)  [unwired: 1 in, 1 out]
                n125 = Enqueue Element(queue=w260, element="clear console", error in (no error)=w262) -> (error out=w261:errorcluster)  [unwired: 1 in, 2 out]
              }
            }
          }
          frame "any input" {
            w275 = "a" ("write buffer")
            n126 = Unbundle By Name(w280) -> ("Console"=w273:refnum<vi>, "COM"=w270:refnum<visa-resource-name>)
            n127 = property class="Str"(reference=w273) -> (reference out=w278:refnum<vi>, error out=w272:errorcluster, "Value"=w279:string)  [unwired: 1 in]
            n128 = VISA Write(VISA resource name=w270, write buffer=w275, error in (no error)=w271) -> (error out=w269:errorcluster)  [unwired: 2 out]
            n129 = Concatenate Strings(w279, ">" ("string"), w275, "\r") -> (w277:string)
            n130 = property class="Str"(reference=w278, error in=w272, "Value"=w277) -> ()  [unwired: 2 out]
            n131 = case shown="No Error" w269 {
              selector: w269 -> [w282 w287]
              tunnel: [w283 w285] -> w268
              tunnel: w267 -> [w281 w286]
              frame No Error {
                n132 = Enqueue Element(queue=w281, element="destroyenv", error in (no error)=w282) -> (error out=w283:errorcluster)  [unwired: 1 in, 2 out]
              }
              frame Error {
                n133 = Enqueue Element(queue=w286, element="init", error in (no error)=w287) -> (error out=w285:errorcluster)  [unwired: 1 in, 2 out]
              }
            }
          }
          frame "destroyenv" {
            n134 = Unbundle By Name(w297) -> ("Console"=w296:refnum<vi>, "COM"=w295:refnum<visa-resource-name>)  [unwired: 1 out]
            n135 = Concatenate Strings(w294, "\r") -> (w292:string)
            n136 = VISA Write(VISA resource name=w295, write buffer=w292) -> (VISA resource name out=w302:refnum<visa-resource-name>, error out=w301:errorcluster)  [unwired: 1 in, 1 out]
            n137 = call "Stall Data Flow.vim"("value in"=w301, "milliseconds to wait"=u32 100) -> ("value out"=w291:errorcluster)  [unwired: 1 out]
            n138 = while {
              shift-right: [w328] -> w299
              shift-left: w302 -> [w322]
              tunnel: [w326] -> w300
              tunnel: w291 -> [w321]
              tunnel: w296 -> [w314]
              stop <- w327 stop-if-true
              # "Serial Write and Read Loop"
              n139 = property class="Str"(reference=w314) -> (reference out=w317:refnum<vi>, "Value"=w313:string)  [unwired: 1 in, 1 out]
              n140 = property class="Instr"(reference=w322, error in=w321) -> (reference out=w320:refnum<visa-resource-name>, error out=w319:errorcluster, "Serial Settings:Number of Bytes at Serial Port"=w318:u32)
              n141 = VISA Read(VISA resource name=w320, byte count=w318, error in (no error)=w319) -> (VISA resource name out=w328:refnum<visa-resource-name>, read buffer=w315:string, error out=w326:errorcluster)  [unwired: 1 out]
              n142 = Concatenate Strings(w313, w315) -> (w316:string)
              n143 = Match Pattern(string=w315, regular expression="done") -> (offset past match=w324:i32)  [unwired: 1 in, 3 out]
              n144 = Greater Or Equal To 0?(x=w324) -> (x >= 0?=w323:bool)
              n145 = property class="Str"(reference=w317, "Value"=w316) -> ()  [unwired: 1 in, 2 out]
              n146 = Or(x=w326, y=w323) -> (x .or. y?=w327:bool)
            }
            n147 = case shown="No Error" w300 {
              selector: w300 -> [w306 w309]
              tunnel: w299 -> [_ w312]
              tunnel: w298 -> [w305 w307]
              tunnel: [w303 w310] -> w289
              frame No Error {
                n148 = Enqueue Element(queue=w305, element="send file", error in (no error)=w306) -> (error out=w303:errorcluster)  [unwired: 1 in, 2 out]
              }
              frame Error {
                n149 = Enqueue Element At Opposite End(queue=w307, element="error", error in (no error)=w309) -> (error out=w308:errorcluster)  [unwired: 1 in, 2 out]
                n150 = VISA Close(VISA resource name=w312, error in (no error)=w308) -> (error out=w310:errorcluster)
              }
            }
          }
          frame "send file" {
            n151 = Unbundle By Name(w351) -> ("Console"=w337:refnum<vi>, "COM"=w341:refnum<visa-resource-name>, "Android path"=w331:path)
            n152 = String To Path(string="gui_env.txt") -> (path=w330:path)
            n153 = Build Path(base path=w331, name or relative path=w330) -> (appended path=w329:path)
            n154 = Open/Create/Replace File(file path (use dialog)=w329, operation (0:open)=T9."open") -> (refnum out=w349:refnum<file>, error out=w347:errorcluster)  [unwired: 4 in, 1 out]
            n155 = Read from Text File(file (use dialog)=w349, error in=w347) -> (text=w345:string, error out=w339:errorcluster)  [unwired: 2 in, 2 out]
            n156 = Spreadsheet String To Array(delimiter (Tab)="\n", format string="%s", spreadsheet string=w345, array type (2D Dbl)=string[] []) -> (array=w342:string[])
            n157 = for {
              tunnel: w342 -> [w355] mode=indexing
              tunnel: w341 -> [w360]
              shift-right: [w356] -> w340
              shift-left: w339 -> [w357]
              stop <- w356 stop-if-true
              n158 = Concatenate Strings(w355, "\r") -> (w354:string)
              n159 = VISA Write(VISA resource name=w360, write buffer=w354, error in (no error)=w357) -> (error out=w359:errorcluster)  [unwired: 2 out]
              n160 = call "Stall Data Flow.vim"("value in"=w359, "milliseconds to wait"=u32 50) -> ("value out"=w356:errorcluster)  [unwired: 1 out]
            }
            n161 = case shown="No Error" w340 {
              selector: w340 -> [w362 w365]
              tunnel: w352 -> [w364 w367]
              tunnel: [w361 w365] -> w338
              frame No Error {
                n162 = Enqueue Element(queue=w364, element="read buffer", error in (no error)=w362) -> (error out=w361:errorcluster)  [unwired: 1 in, 2 out]
              }
              frame Error {
                n163 = Enqueue Element At Opposite End(queue=w367, element="error") -> ()  [unwired: 2 in, 3 out]
              }
            }
            n164 = property class="Str"(reference=w337) -> (reference out=w336:refnum<vi>, "Value"=w335:string)  [unwired: 1 in, 1 out]
            n165 = Concatenate Strings(w335, "\r") -> (w334:string)
            n166 = property class="Str"(reference=w336, "Value"=w334) -> ()  [unwired: 1 in, 2 out]
          }
          frame "read buffer" {
            n167 = Unbundle By Name(w371) -> ("Console"=w368:refnum<vi>, "COM"=w372:refnum<visa-resource-name>)
            n168 = while {
              tunnel: [w382] -> w375
              tunnel: w372 -> [w381]
              tunnel: w368 -> [w376]
              stop <- w386 stop-if-true
              n169 = property class="Instr"(reference=w381) -> (reference out=w387:refnum<visa-resource-name>, error out=w385:errorcluster, "Serial Settings:Number of Bytes at Serial Port"=w383:u32)  [unwired: 1 in]
              n170 = Equal To 0?(x=w383) -> (x = 0?=w384:bool)
              n171 = case shown="False" w384 {
                tunnel: w387 -> [w392 _]
                tunnel: w385 -> [w391 w393]
                tunnel: [w390 w393] -> w382
                tunnel: w383 -> [w389 _]
                tunnel: [w388 _] -> w379
                frame False {
                  n172 = VISA Read(VISA resource name=w392, byte count=w389, error in (no error)=w391) -> (read buffer=w388:string, error out=w390:errorcluster)  [unwired: 2 out]
                }
                frame True {
                }
              }
              n173 = Or(x=w382, y=w384) -> (x .or. y?=w386:bool)
              n174 = property class="Str"(reference=w376) -> (reference out=w377:refnum<vi>, "Value"=w380:string)  [unwired: 1 in, 1 out]
              n175 = Concatenate Strings(w380, w379) -> (w378:string)
              n176 = property class="Str"(reference=w377, "Value"=w378) -> ()  [unwired: 1 in, 2 out]
            }
            n177 = Enqueue Element(queue=w374, element="saveenv", error in (no error)=w375) -> (error out=w369:errorcluster)  [unwired: 1 in, 2 out]
          }
          frame "saveenv" {
            n178 = Unbundle By Name(w395) -> ("Console"=w400:refnum<vi>, "COM"=w402:refnum<visa-resource-name>)  [unwired: 1 out]
            n179 = Concatenate Strings("\r", w398, "\r") -> (w399:string)
            n180 = VISA Write(VISA resource name=w402, write buffer=w399) -> (VISA resource name out=w406:refnum<visa-resource-name>, error out=w405:errorcluster)  [unwired: 1 in, 1 out]
            n181 = while {
              shift-right: [w445] -> w403
              shift-left: w406 -> [w439]
              tunnel: [w443] -> w404
              tunnel: w405 -> [w438]
              tunnel: w400 -> [w430]
              stop <- w444 stop-if-true
              # "Serial Write and Read Loop"
              n182 = property class="Instr"(reference=w439, error in=w438) -> (reference out=w437:refnum<visa-resource-name>, error out=w436:errorcluster, "Serial Settings:Number of Bytes at Serial Port"=w435:u32)
              n183 = property class="Str"(reference=w430) -> (reference out=w434:refnum<vi>, "Value"=w432:string)  [unwired: 1 in, 1 out]
              n184 = VISA Read(VISA resource name=w437, byte count=w435, error in (no error)=w436) -> (VISA resource name out=w445:refnum<visa-resource-name>, read buffer=w431:string, error out=w443:errorcluster)  [unwired: 1 out]
              n185 = Concatenate Strings(w432, w431) -> (w433:string)
              n186 = Match Pattern(string=w431, regular expression="done") -> (offset past match=w441:i32)  [unwired: 1 in, 3 out]
              n187 = property class="Str"(reference=w434, "Value"=w433) -> (reference out=w429:refnum<vi>, error out=w427:errorcluster)  [unwired: 1 in]
              n188 = Greater Or Equal To 0?(x=w441) -> (x >= 0?=w440:bool)
              n189 = property class="Str"(reference=w429, error in=w427, "Text.Scroll Position"=u32 4294967295) -> ()  [unwired: 2 out]
              n190 = Or(x=w443, y=w440) -> (x .or. y?=w444:bool)
            }
            n191 = case shown="No Error" w404 {
              selector: w404 -> [w421 w424]
              tunnel: w403 -> [_ _]
              tunnel: w401 -> [w420 w425]
              tunnel: [w412 w423] -> w396
              frame No Error {
                n192 = Enqueue Element(queue=w420, element="flush", error in (no error)=w421) -> (queue out=w414:refnum<queue>, error out=w415:errorcluster)  [unwired: 1 in, 1 out]
                n193 = Enqueue Element(queue=w414, element="close visa", error in (no error)=w415) -> (queue out=w418:refnum<queue>, error out=w409:errorcluster)  [unwired: 1 in, 1 out]
                n194 = Enqueue Element(queue=w418, element="clear console", error in (no error)=w409) -> (queue out=w410:refnum<queue>, error out=w408:errorcluster)  [unwired: 1 in, 1 out]
                n195 = Enqueue Element(queue=w410, element="reboot", error in (no error)=w408) -> (queue out=w416:refnum<queue>, error out=w417:errorcluster)  [unwired: 1 in, 1 out]
                n196 = Enqueue Element(queue=w416, element="prepare gui", error in (no error)=w417) -> (error out=w412:errorcluster)  [unwired: 1 in, 2 out]
              }
              frame Error {
                n197 = Enqueue Element At Opposite End(queue=w425, element="error", error in (no error)=w424) -> (error out=w423:errorcluster)  [unwired: 1 in, 2 out]
              }
            }
          }
          frame "reboot" {
            n198 = Unbundle By Name(w455) -> ("Console"=w449:refnum<vi>, "IO task"=w454:refnum<k24>)
            n199 = disable-structure shown="Disabled" {
              disable-tunnel: w454 -> [w457 _]
              disable-tunnel: w447 -> [_ w474]
              disable-tunnel: [_ w473] -> w446
              frame Disabled {
                n200 = flat-sequence {
                  tunnel: w457 -> [w465]
                  tunnel: [w463] -> w461
                  tunnel: [w462] -> w460
                  tunnel: w461 -> [w468]
                  tunnel: [w468] -> w459
                  tunnel: w460 -> [w466]
                  tunnel: [w466] -> w458
                  tunnel: w459 -> [w471]
                  tunnel: w458 -> [w469]
                  frame #0 {
                    # "turn off display"
                    n201 = call-poly <vilib>:"ULx Write.vi"("task in"=w465, "data"=FALSE) -> ("task out"=w463:refnum<k24>, "error out"=w462:errorcluster)  [unwired: 11 in, 1 out]
                  }
                  frame #1 {
                    n202 = Wait (ms)(milliseconds to wait=u32 500) -> ()  [unwired: 1 out]
                  }
                  frame #2 {
                    # "turn on the display"
                    n203 = call-poly <vilib>:"ULx Write.vi"("task in"=w471, "data"=TRUE, "error in"=w469) -> ()  [unwired: 10 in, 3 out]
                  }
                  frame #3 {
                    n204 = Wait (ms)(milliseconds to wait=u32 500) -> ()  [unwired: 1 out]
                  }
                  frame #4 {
                  }
                }
              }
              frame Enabled {
                n205 = Two Button Dialog(message="reinicia el monitor!", 1:"Abort!" ("F button name (\"Cancel\")"), 2:"Reiniciado" ("T button name (\"OK\")")) -> (T button?=w475:bool)
                n206 = case shown="False" w475 {
                  tunnel: w474 -> [w481 _]
                  tunnel: [w480 _] -> w473
                  frame False {
                    n207 = Enqueue Element At Opposite End(queue=w481, element="error") -> (error out=w480:errorcluster)  [unwired: 2 in, 2 out]
                  }
                  frame True {
                  }
                }
              }
            }
            n208 = property class="Str"(reference=w449) -> (reference out=w453:refnum<vi>, "Value"=w451:string)  [unwired: 1 in, 1 out]
            n209 = Concatenate Strings(w451, "\r", "\nRE-BOOTING...\n" ("string")) -> (w452:string)
            n210 = property class="Str"(reference=w453, "Value"=w452) -> ()  [unwired: 1 in, 2 out]
          }
          frame "close visa" {
            n211 = Unbundle By Name(w489) -> ("COM"=w482:refnum<visa-resource-name>)
            n212 = VISA Clear(VISA resource name=w482) -> (VISA resource name out=w483:refnum<visa-resource-name>, error out=w484:errorcluster)  [unwired: 1 in]
            n213 = VISA Close(VISA resource name=w483, error in (no error)=w484) -> (error out=w485:errorcluster)
            n214 = Bundle By Name(cluster=w489, "COM"=refnum<visa-resource-name> refnum) -> (w488:T2)
          }
          frame "clear console" {
            n215 = Unbundle By Name(w492) -> ("Console"=w491:refnum<vi>)
            n216 = property class="Str"(reference=w491, "Value"="\n   Ouset_Medical®\n\n") -> ()  [unwired: 1 in, 2 out]
          }
          frame "prepare gui" {
            n217 = Unbundle By Name(w494) -> ("Console"=w504:refnum<vi>)
            n218 = property class="Str"(reference=w504) -> (reference out=w503:refnum<vi>, "Value"=w501:string)  [unwired: 1 in, 1 out]
            n219 = Unbundle By Name(w494) -> ("Android path"=w514:path)
            n220 = call "Progress bar v2.vi"("TIme (s)"=310.0, "Title"="Preparing GUI") -> ()  [unwired: 9 in, 1 out]
            n221 = Concatenate Strings(w501, "\n>Preparing the GUI...\n" ("Value")) -> (w502:string)
            n222 = property class="Str"(reference=w503, "Value"=w502) -> (reference out=w505:refnum<vi>)  [unwired: 1 in, 1 out]
            n223 = call <vilib>:"System Exec.vi"("run minimized? (F)"=TRUE, "working directory"=w514, "command line"="python prepare_gui_board.py") -> ("standard error"=w515:string, "standard output"=w513:string)  [unwired: 5 in, 2 out]
            n224 = property class="Str"(reference=w505) -> (reference out=w518:refnum<vi>, "Value"=w519:string)  [unwired: 1 in, 1 out]
            n225 = Concatenate Strings(w519, w513, w515) -> (w517:string)
            n226 = property class="Str"(reference=w518, "Value"=w517) -> (reference out=w499:refnum<vi>, error out=w498:errorcluster)  [unwired: 1 in]
            n227 = Match Pattern(string=w513, regular expression="Watch display and make sure Tablo logo appears after a few minutes.") -> (offset past match=w511:i32)  [unwired: 1 in, 3 out]
            n228 = Greater Or Equal To 0?(x=w511) -> (x >= 0?=w509:bool)
            n229 = property class="Str"(reference=w499, error in=w498, "Text.Scroll Position"=u32 4294967295) -> ()  [unwired: 2 out]
            n230 = case shown="True" w509 {
              tunnel: w510 -> [w524 w531]
              tunnel: w508 -> [w521 w526]
              tunnel: [w522 w530] -> w506
              frame False {
                n231 = flat-sequence {
                  frame #0 {
                    n232 = call <vilib>:"Close Progress Bar.vi"() -> ()  [unwired: 10 in, 2 out]
                  }
                  frame #1 {
                    n233 = One Button Dialog(message="--------------------------------------------\nError occurred while connecting to \nthe GUI board\n--------------------------------------------") -> ()  [unwired: 1 in, 1 out]
                  }
                }
                n234 = Enqueue Element At Opposite End(queue=w524, element="error", error in (no error)=w521) -> (error out=w522:errorcluster)  [unwired: 1 in, 2 out]
              }
              frame True {
                n235 = call <vilib>:"Close Progress Bar.vi"() -> ()  [unwired: 10 in, 2 out]
                n236 = Enqueue Element(queue=w531, element="clear console", error in (no error)=w526) -> (queue out=w529:refnum<queue>, error out=w527:errorcluster)  [unwired: 1 in, 1 out]
                n237 = Enqueue Element(queue=w529, element="adb version", error in (no error)=w527) -> (error out=w530:errorcluster)  [unwired: 1 in, 2 out]
              }
            }
          }
          frame "adb version" {
            w549 = "1.0.36"  # adb target version
            n238 = Unbundle By Name(w555) -> ("Console"=w542:refnum<vi>, "Version path"=w534:path)
            n239 = property class="Str"(reference=w542) -> (reference out=w538:refnum<vi>, "Value"=w541:string)  [unwired: 1 in, 1 out]
            n240 = Concatenate Strings(w541, ">" ("string"), w539, "\r") -> (w536:string)
            n241 = property class="Str"(reference=w538, "Value"=w536) -> (reference out=w537:refnum<vi>)  [unwired: 1 in, 1 out]
            n242 = call <vilib>:"System Exec.vi"("run minimized? (F)"=TRUE, "working directory"=w534, "command line"=w539) -> ("standard error"=w545:string, "standard output"=w550:string)  [unwired: 5 in, 2 out]
            n243 = property class="Str"(reference=w537) -> (reference out=w554:refnum<vi>, error out=w551:errorcluster, "Value"=w553:string)  [unwired: 1 in]
            n244 = Match Pattern(string=w550, regular expression=w549) -> (offset past match=w548:i32)  [unwired: 1 in, 3 out]
            n245 = Concatenate Strings(w553, w550, w545) -> (w552:string)
            n246 = Greater Or Equal To 0?(x=w548) -> (x >= 0?=w547:bool)
            n247 = property class="Str"(reference=w554, error in=w551, "Value"=w552) -> ()  [unwired: 2 out]
            n248 = case shown="False" w547 {
              tunnel: w546 -> [w560 w573]
              tunnel: w544 -> [w556 w571]
              tunnel: [w557 w565] -> w543
              frame False {
                n249 = One Button Dialog(message="Error: \n incorrect Android Debug Bridge (ADB) version\n\nMake sure you have installed the 1.0.36 version\nand try again.") -> ()  [unwired: 1 in, 1 out]
                n250 = Enqueue Element At Opposite End(queue=w560, element="error", error in (no error)=w556) -> (error out=w557:errorcluster)  [unwired: 1 in, 2 out]
              }
              frame True {
                (unwired) "os build" ("element")
                n251 = Enqueue Element(queue=w573, element="reboot", error in (no error)=w571) -> (queue out=w575:refnum<queue>, error out=w572:errorcluster)  [unwired: 1 in, 1 out]
                n252 = Enqueue Element(queue=w575, element="delay", error in (no error)=w572) -> (queue out=w568:refnum<queue>, error out=w570:errorcluster)  [unwired: 1 in, 1 out]
                n253 = Enqueue Element(queue=w568, element="adb connect", error in (no error)=w570) -> (queue out=w566:refnum<queue>, error out=w562:errorcluster)  [unwired: 1 in, 1 out]
                n254 = Enqueue Element(queue=w566, element="clear console", error in (no error)=w562) -> (queue out=w564:refnum<queue>, error out=w561:errorcluster)  [unwired: 1 in, 1 out]
                n255 = Enqueue Element(queue=w564, element="check screen", error in (no error)=w561) -> (error out=w565:errorcluster)  [unwired: 1 in, 2 out]
              }
            }
          }
          frame "IPv4" {
            n256 = Unbundle By Name(w581) -> ("Console"=w577:refnum<vi>, "COM"=w579:refnum<visa-resource-name>)
            n257 = while {
              shift-right: [w606] -> _
              shift-left: w579 -> [w603]
              tunnel: [w605] -> w580
              tunnel: [w599] -> w582
              tunnel: w577 -> [w585]
              i -> [w594]
              stop <- w597 stop-if-true
              # "Serial Write and Read Loop"
              n258 = property class="Instr"(reference=w603) -> (reference out=w602:refnum<visa-resource-name>, error out=w601:errorcluster, "Serial Settings:Number of Bytes at Serial Port"=w600:u32)  [unwired: 1 in]
              n259 = property class="Str"(reference=w585) -> (reference out=w592:refnum<vi>, "Value"=w589:string)  [unwired: 1 in, 1 out]
              n260 = Equal To 0?(x=w594) -> (x = 0?=w593:bool)
              n261 = VISA Read(VISA resource name=w602, byte count=w600, error in (no error)=w601) -> (VISA resource name out=w606:refnum<visa-resource-name>, read buffer=w588:string, error out=w605:errorcluster)  [unwired: 1 out]
              n262 = Concatenate Strings(w589, w588) -> (w590:string)
              n263 = call "Elapsed Time"("Time Target (s)"=60.0, "Reset"=w593) -> ("Time has Elapsed"=w596:bool)  [unwired: 10 in, 7 out]
              n264 = property class="Str"(reference=w592, "Value"=w590) -> (reference out=w587:refnum<vi>)  [unwired: 1 in, 1 out]
              n265 = Match Pattern(string=w588, regular expression="link becomes ready") -> (offset past match=w604:i32)  [unwired: 1 in, 3 out]
              n266 = Greater Or Equal To 0?(x=w604) -> (x >= 0?=w599:bool)
              n267 = property class="Str"(reference=w587, "Text.Scroll Position"=u32 4294967295) -> ()  [unwired: 1 in, 2 out]
              n268 = Or(x=w605, y=w599) -> (x .or. y?=w598:bool)
              n269 = Or(x=w598, y=w596) -> (x .or. y?=w597:bool)
            }
            n270 = case shown="False" w582 {
              tunnel: w584 -> [w610 w614]
              tunnel: w580 -> [w608 w615]
              tunnel: [w607 w611] -> w578
              frame False {
                n271 = Enqueue Element At Opposite End(queue=w610, element="error", error in (no error)=w608) -> (error out=w607:errorcluster)  [unwired: 1 in, 2 out]
              }
              frame True {
                n272 = Enqueue Element At Opposite End(queue=w614, element="flush", error in (no error)=w615) -> (queue out=w612:refnum<queue>, error out=w613:errorcluster)  [unwired: 1 in, 1 out]
                n273 = Enqueue Element(queue=w612, element="clear console", error in (no error)=w613) -> (error out=w611:errorcluster)  [unwired: 1 in, 2 out]
              }
            }
          }
          frame "adb connect" {
            n274 = Unbundle By Name(w620) -> ("Console"=w625:refnum<vi>, "Version path"=w618:path)
            n275 = property class="Str"(reference=w625) -> (reference out=w626:refnum<vi>, "Value"=w624:string)  [unwired: 1 in, 1 out]
            n276 = Concatenate Strings(w624, "\n>Connecting to GUI board...\n") -> (w623:string)
            n277 = property class="Str"(reference=w626, "Value"=w623) -> (reference out=w621:refnum<vi>)  [unwired: 1 in, 1 out]
            n278 = call <vilib>:"System Exec.vi"("run minimized? (F)"=TRUE, "working directory"=w618, "command line"="adb connect 10.134.246.252") -> ("standard error"=w629:string, "standard output"=w637:string)  [unwired: 5 in, 2 out]
            n279 = property class="Str"(reference=w621) -> (reference out=w641:refnum<vi>, error out=w638:errorcluster, "Value"=w640:string)  [unwired: 1 in]
            n280 = Concatenate Strings(w640, w637, w629) -> (w639:string)
            n281 = Match Pattern(string=w637, regular expression="connected") -> (offset past match=w635:i32)  [unwired: 1 in, 3 out]
            n282 = Greater Or Equal To 0?(x=w635) -> (x >= 0?=w634:bool)
            n283 = property class="Str"(reference=w641, error in=w638, "Value"=w639) -> ()  [unwired: 2 out]
            n284 = case shown="False" w634 {
              tunnel: w633 -> [w649 _]
              tunnel: [w648 w661] -> w628
              tunnel: w627 -> [w647 w661]
              tunnel: w620 -> [w645 w660]
              tunnel: [w644 w660] -> w619
              frame False {
                n285 = Unbundle By Name(w645) -> ("Attempts left"=w643:i32)
                n286 = Less Or Equal To 0?(x=w643) -> (x <= 0?=w646:bool)
                n287 = Decrement(x=w643) -> (x-1=w642:i32)
                n288 = case shown="False" w646 {
                  tunnel: w649 -> [w655 w658]
                  tunnel: [w654 w657] -> w648
                  tunnel: w647 -> [w653 w656]
                  frame False {
                    n289 = call "Stall Data Flow.vim"("value in"=w653, "milliseconds to wait"=u32 1000) -> ("value out"=w651:errorcluster)  [unwired: 1 out]
                    n290 = Enqueue Element At Opposite End(queue=w655, element="adb connect", error in (no error)=w651) -> (error out=w654:errorcluster)  [unwired: 1 in, 2 out]
                  }
                  frame True {
                    n291 = Enqueue Element At Opposite End(queue=w658, element="unable to connect", error in (no error)=w656) -> (error out=w657:errorcluster)  [unwired: 1 in, 2 out]
                  }
                }
                n292 = Bundle By Name(cluster=w645, "Attempts left"=w642) -> (w644:T2)
              }
              frame True {
              }
            }
          }
          frame "unable to connect" {
            n293 = Two Button Dialog(message="--------------------------------------\nError:\nUnable to connect to 10.134.246.252!\n--------------------------------------\nCheck the ethernet connection,\nreboot & try again.", 1:"Stop" ("F button name (\"Cancel\")"), 2:"Try again" ("T button name (\"OK\")")) -> (T button?=w665:bool)
            n294 = case shown="True" w665 {
              tunnel: w664 -> [w672 w675]
              tunnel: [w670 w674] -> w663
              frame False {
                n295 = Enqueue Element At Opposite End(queue=w672, element="error") -> (error out=w670:errorcluster)  [unwired: 2 in, 2 out]
              }
              frame True {
                n296 = Enqueue Element At Opposite End(queue=w675, element="adb connect") -> (error out=w674:errorcluster)  [unwired: 2 in, 2 out]
              }
            }
          }
          frame "os build" {
            n297 = Unbundle By Name(w701) -> ("Console"=w681:refnum<vi>, "Version path"=w676:path)
            n298 = property class="Str"(reference=w681) -> (reference out=w684:refnum<vi>, error out=w682:errorcluster, "Value"=w683:string)  [unwired: 1 in]
            n299 = Concatenate Strings(w683, ">adb shell cat/system/build.prop\n") -> (w680:string)
            n300 = property class="Str"(reference=w684, error in=w682, "Value"=w680) -> (reference out=w679:refnum<vi>)  [unwired: 1 out]
            n301 = call <vilib>:"System Exec.vi"("run minimized? (F)"=TRUE, "working directory"=w676, "command line"="adb shell cat/system/build.prop") -> ("standard error"=w689:string, "standard output"=w696:string)  [unwired: 5 in, 2 out]
            n302 = property class="Str"(reference=w679) -> (reference out=w700:refnum<vi>, error out=w697:errorcluster, "Value"=w699:string)  [unwired: 1 in]
            n303 = Concatenate Strings(w699, w696, w689) -> (w698:string)
            n304 = Match Pattern(string=w696, regular expression="ouset.osbuild=4.0.0.3") -> (offset past match=w694:i32)  [unwired: 1 in, 3 out]
            n305 = Greater Or Equal To 0?(x=w694) -> (x >= 0?=w693:bool)
            n306 = property class="Str"(reference=w700, error in=w697, "Value"=w698) -> (reference out=w686:refnum<vi>)  [unwired: 1 out]
            n307 = case shown="False" w693 {
              tunnel: w692 -> [w704 w711]
              tunnel: [w703 w709] -> w688
              tunnel: w687 -> [w702 w707]
              frame False {
                n308 = One Button Dialog(message="Error: \nincorrect GUI Operative System version \n\nMake sure the OS build is the 4.0.0.3\n& try again") -> ()  [unwired: 1 in, 1 out]
                n309 = Enqueue Element(queue=w704, element="error", error in (no error)=w702) -> (error out=w703:errorcluster)  [unwired: 1 in, 2 out]
              }
              frame True {
                n310 = Enqueue Element(queue=w711, element="clear console", error in (no error)=w707) -> (queue out=w712:refnum<queue>, error out=w708:errorcluster)  [unwired: 1 in, 1 out]
                n311 = Enqueue Element(queue=w712, element="check screen", error in (no error)=w708) -> (error out=w709:errorcluster)  [unwired: 1 in, 2 out]
              }
            }
            n312 = property class="Str"(reference=w686, "Text.Scroll Position"=u32 4294967295) -> ()  [unwired: 1 in, 2 out]
          }
          frame "check screen" {
            n313 = Two Button Dialog(message="Realice la siguiente verificación funcional de la pantalla táctil, toque cada esquina \ny verifique que aparecen los siguientes números en cada una de ellas:\n-superior izquierda: 0 (+40 / -0), 0 (+40 / -0)\n-inferior izquierda: 0 (+40 / -0), 768 (+0 / -40)\n-inferior derecha: 1024 (+0 / -40), 768 (+0 / -40)\n-superior derecha: 1024 (+0 / -40), 0 (+40 / -0)\nEl numero aparece en la parte inferior central de la pantalla en cada caso. \nSi el número no coincide favor de comunicarse con el supervisor o el ingeniero.", 1:"¡Abortar!" ("F button name (\"Cancel\")"), 2:"Todo bien" ("T button name (\"OK\")")) -> (T button?=w718:bool)
            n314 = case shown="True" w718 {
              tunnel: w717 -> [w726 w729]
              tunnel: [w724 w728] -> w715
              tunnel: w714 -> [w723 w727]
              frame False {
                n315 = Enqueue Element(queue=w726, element="error", error in (no error)=w723) -> (error out=w724:errorcluster)  [unwired: 1 in, 2 out]
              }
              frame True {
                n316 = Enqueue Element(queue=w729, element="adb uninstall", error in (no error)=w727) -> (error out=w728:errorcluster)  [unwired: 1 in, 2 out]
              }
            }
          }
          frame "adb uninstall" {
            n317 = Unbundle By Name(w756) -> ("Console"=w737:refnum<vi>, "Version path"=w731:path)
            n318 = property class="Str"(reference=w737) -> (reference out=w738:refnum<vi>, "Value"=w736:string)  [unwired: 1 in, 1 out]
            n319 = Concatenate Strings(w736, "\n>adb uninstall sequoia.gui.demo\n") -> (w734:string)
            n320 = property class="Str"(reference=w738, "Value"=w734) -> (reference out=w735:refnum<vi>)  [unwired: 1 in, 1 out]
            n321 = call <vilib>:"System Exec.vi"("run minimized? (F)"=TRUE, "working directory"=w731, "command line"="adb uninstall sequoia.gui.demo") -> ("standard error"=w743:string, "standard output"=w751:string)  [unwired: 5 in, 2 out]
            n322 = property class="Str"(reference=w735) -> (reference out=w755:refnum<vi>, error out=w752:errorcluster, "Value"=w754:string)  [unwired: 1 in]
            n323 = Concatenate Strings(w754, w751, w743) -> (w753:string)
            n324 = Match Pattern(string=w751, regular expression="Success") -> (offset past match=w750:i32)  [unwired: 1 in, 3 out]
            n325 = Match Pattern(string=w743, regular expression="kill-server") -> (offset past match=w742:i32)  [unwired: 1 in, 3 out]
            n326 = Greater Or Equal To 0?(x=w750) -> (x >= 0?=w749:bool)
            n327 = Greater Or Equal To 0?(x=w742) -> (x >= 0?=w741:bool)
            n328 = property class="Str"(reference=w755, error in=w752, "Value"=w753) -> ()  [unwired: 2 out]
            n329 = case shown="True" w749 {
              tunnel: w748 -> [w760 w776]
              tunnel: w741 -> [w759 _]
              tunnel: [w758 w772] -> w740
              tunnel: w739 -> [w757 w771]
              frame False {
                n330 = case shown="True" w759 {
                  tunnel: w760 -> [w764 w770]
                  tunnel: [w762 w768] -> w758
                  tunnel: w757 -> [w761 w767]
                  frame False {
                    n331 = One Button Dialog(message="------------------------------\nError: unhandle excepcion in\nadb uninstall\n------------------------------", button name ("OK")="Abort") -> ()  [unwired: 1 out]
                    n332 = Enqueue Element(queue=w764, element="error", error in (no error)=w761) -> (error out=w762:errorcluster)  [unwired: 1 in, 2 out]
                  }
                  frame True {
                    n333 = Enqueue Element(queue=w770, element="adb kill-server", error in (no error)=w767) -> (error out=w768:errorcluster)  [unwired: 1 in, 2 out]
                  }
                }
              }
              frame True {
                n334 = call "Stall Data Flow.vim"("value in"=w776, "milliseconds to wait"=u32 1000) -> ("value out"=w774:refnum<queue>)  [unwired: 1 out]
                n335 = Enqueue Element(queue=w774, element="adb install", error in (no error)=w771) -> (error out=w772:errorcluster)  [unwired: 1 in, 2 out]
              }
            }
          }
          frame "adb kill-server" {
            (unwired) enum16{"Open", "Write", "Read", "Close"}."Read" ("Operation")
            n336 = Unbundle By Name(w798) -> ("Console"=w792:refnum<vi>, "Version path"=w777:path)
            n337 = property class="Str"(reference=w792) -> (reference out=w791:refnum<vi>, "Value"=w790:string)  [unwired: 1 in, 1 out]
            n338 = Concatenate Strings(w790, "\n>adb kill-server\n") -> (w789:string)
            n339 = property class="Str"(reference=w791, "Value"=w789) -> (reference out=w787:refnum<vi>)  [unwired: 1 in, 1 out]
            n340 = call <vilib>:"System Exec.vi"("run minimized? (F)"=TRUE, "working directory"=w777, "command line"=w795) -> ("standard error"=w799:string, "standard output"=w800:string)  [unwired: 5 in, 2 out]
            n341 = property class="Str"(reference=w787) -> (reference out=w804:refnum<vi>, error out=w801:errorcluster, "Value"=w803:string)  [unwired: 1 in]
            n342 = Concatenate Strings(w803, w800, w799) -> (w802:string)
            n343 = property class="Str"(reference=w804, error in=w801, "Value"=w802) -> (error out=w794:errorcluster)  [unwired: 1 out]
            n344 = call "Stall Data Flow.vim"("value in"=w794, "milliseconds to wait"=u32 1000) -> ("value out"=w780:errorcluster)  [unwired: 1 out]
            n345 = Enqueue Element(queue=w797, element="clear console", error in (no error)=w780) -> (queue out=w782:refnum<queue>, error out=w781:errorcluster)  [unwired: 1 in, 1 out]
            n346 = Enqueue Element(queue=w782, element="adb connect", error in (no error)=w781) -> (queue out=w784:refnum<queue>, error out=w786:errorcluster)  [unwired: 1 in, 1 out]
            n347 = Enqueue Element(queue=w784, element="adb uninstall", error in (no error)=w786) -> (error out=w785:errorcluster)  [unwired: 1 in, 2 out]
          }
          frame "adb install" {
            n348 = Unbundle By Name(w828) -> ("Console"=w813:refnum<vi>, "Version path"=w805:path)
            n349 = property class="Str"(reference=w813) -> (reference out=w814:refnum<vi>, "Value"=w810:string)  [unwired: 1 in, 1 out]
            n350 = Concatenate Strings(w810, "\n>adb install -r SequoiaGUI.apk\n") -> (w811:string)
            n351 = property class="Str"(reference=w814, "Value"=w811) -> (reference out=w812:refnum<vi>)  [unwired: 1 in, 1 out]
            n352 = call <vilib>:"System Exec.vi"("run minimized? (F)"=TRUE, "working directory"=w805, "command line"="adb install -r SequoiaGUI.apk") -> ("standard error"=w816:string, "standard output"=w823:string)  [unwired: 5 in, 2 out]
            n353 = property class="Str"(reference=w812) -> (reference out=w827:refnum<vi>, error out=w824:errorcluster, "Value"=w826:string)  [unwired: 1 in]
            n354 = Concatenate Strings(w826, w823, w816) -> (w825:string)
            n355 = Match Pattern(string=w823, regular expression="Success") -> (offset past match=w821:i32)  [unwired: 1 in, 3 out]
            n356 = Greater Or Equal To 0?(x=w821) -> (x >= 0?=w820:bool)
            n357 = property class="Str"(reference=w827, error in=w824, "Value"=w825) -> (reference out=w806:refnum<vi>)  [unwired: 1 out]
            n358 = case shown="False" w820 {
              tunnel: w819 -> [w832 w838]
              tunnel: [w830 w834] -> w815
              frame False {
                n359 = One Button Dialog(message="------------------------------\nError: unhandle excepcion in\nadb uninstall\n------------------------------", button name ("OK")="Abort") -> ()  [unwired: 1 out]
                n360 = Enqueue Element(queue=w832, element="error") -> (error out=w830:errorcluster)  [unwired: 2 in, 2 out]
              }
              frame True {
                n361 = call "Stall Data Flow.vim"("value in"=w838, "milliseconds to wait"=u32 500) -> ("value out"=w836:refnum<queue>)  [unwired: 1 out]
                n362 = Enqueue Element(queue=w836, element="adb reboot") -> (error out=w834:errorcluster)  [unwired: 2 in, 2 out]
              }
            }
            n363 = property class="Str"(reference=w806, "Text.Scroll Position"=u32 4294967295) -> ()  [unwired: 1 in, 2 out]
          }
          frame "adb reboot" {
            n364 = Unbundle By Name(w869) -> ("Console"=w846:refnum<vi>, "Version path"=w839:path)
            n365 = property class="Str"(reference=w846) -> (reference out=w848:refnum<vi>, error out=w849:errorcluster, "Value"=w845:string)  [unwired: 1 in]
            n366 = Concatenate Strings(w845, "\n>adb reboot\n" ("string")) -> (w844:string)
            n367 = property class="Str"(reference=w848, error in=w849, "Value"=w844) -> (reference out=w847:refnum<vi>)  [unwired: 1 out]
            n368 = call <vilib>:"System Exec.vi"("run minimized? (F)"=TRUE, "working directory"=w839, "command line"=w862) -> ("error out"=w857:errorcluster, "standard error"=w860:string, "standard output"=w861:string)  [unwired: 5 in, 1 out]
            n369 = property class="Str"(reference=w847) -> (reference out=w868:refnum<vi>, error out=w865:errorcluster, "Value"=w867:string)  [unwired: 1 in]
            n370 = call "Stall Data Flow.vim"("value in"=w857, "milliseconds to wait"=u32 1000) -> ("value out"=w856:errorcluster)  [unwired: 1 out]
            n371 = Concatenate Strings(w867, w861, w860) -> (w866:string)
            n372 = property class="Str"(reference=w868, error in=w865, "Value"=w866) -> ()  [unwired: 2 out]
            n373 = Enqueue Element(queue=w864, element="clear console") -> (queue out=w842:refnum<queue>)  [unwired: 2 in, 2 out]
            n374 = Enqueue Element(queue=w842, element="reboot", error in (no error)=w856) -> (queue out=w859:refnum<queue>, error out=w854:errorcluster)  [unwired: 1 in, 1 out]
            n375 = Enqueue Element(queue=w859, element="delay", error in (no error)=w854) -> (queue out=w853:refnum<queue>, error out=w851:errorcluster)  [unwired: 1 in, 1 out]
            n376 = Enqueue Element(queue=w853, element="update media", error in (no error)=w851) -> (error out=w850:errorcluster)  [unwired: 1 in, 2 out]
          }
          frame "delay" {
            w872 = "\r"
            n377 = Unbundle By Name(w877) -> ("Console"=w876:refnum<vi>)
            n378 = property class="Str"(reference=w876) -> (reference out=w875:refnum<vi>, "Value"=w873:string)  [unwired: 1 in, 1 out]
            n379 = Concatenate Strings(w873, w872, w872, "." ("string")) -> (w874:string)
            n380 = property class="Str"(reference=w875, "Value"=w874) -> (reference out=w870:refnum<vi>)  [unwired: 1 in, 1 out]
            n381 = for {
              N: 16 -> [_]
              shift-right: [w888] -> w878
              shift-left: w879 -> [w889]
              tunnel: w870 -> [w884]
              n382 = property class="Str"(reference=w884) -> (reference out=w886:refnum<vi>, "Value"=w885:string)  [unwired: 1 in, 1 out]
              n383 = call "Stall Data Flow.vim"("value in"=w889, "milliseconds to wait"=u32 500) -> ("value out"=w888:errorcluster)  [unwired: 1 out]
              n384 = Concatenate Strings(w885, "...") -> (w882:string)
              n385 = property class="Str"(reference=w886, "Value"=w882) -> ()  [unwired: 1 in, 2 out]
            }
          }
          frame "update media" {
            n386 = Unbundle By Name(w899) -> ("Console"=w906:refnum<vi>, "Python 2.7"=w890:path)
            n387 = Open Python Session(python version="2.7.11" ("Python version"), python path=w890, 3:w897) -> (session out=w896:refnum<k35>, error out=w895:errorcluster)
            n388 = property class="Str"(reference=w906) -> (reference out=w905:refnum<vi>, error out=w902:errorcluster, "Value"=w904:string)  [unwired: 1 in]
            n389 = Concatenate Strings(w904, "\n>Opening Update_Media_Labview.py session...") -> (w903:string)
            n390 = property class="Str"(reference=w905, error in=w902, "Value"=w903) -> (reference out=w891:refnum<vi>)  [unwired: 1 out]
            n391 = case shown="No Error" w895 {
              selector: w895 -> [w915 w919]
              tunnel: w894 -> [w916 w920]
              tunnel: [w913 w918] -> w893
              tunnel: w891 -> [w908 _]
              frame No Error {
                n392 = property class="Str"(reference=w908) -> (reference out=w912:refnum<vi>, error out=w909:errorcluster, "Value"=w911:string)  [unwired: 1 in]
                n393 = Concatenate Strings(w911, "\nOK" ("string")) -> (w910:string)
                n394 = Enqueue Element(queue=w916, element="ensure temp dir", error in (no error)=w915) -> (error out=w913:errorcluster)  [unwired: 1 in, 2 out]
                n395 = property class="Str"(reference=w912, error in=w909, "Value"=w910) -> ()  [unwired: 2 out]
              }
              frame Error {
                n396 = One Button Dialog(message="------------------------------------\nFatal error opening python session\n------------------------------------\nPlease check if you have \nthe correct python installed") -> ()  [unwired: 1 in, 1 out]
                n397 = Enqueue Element(queue=w920, element="error", error in (no error)=w919) -> (error out=w918:errorcluster)  [unwired: 1 in, 2 out]
              }
            }
            n398 = Bundle By Name(cluster=w899, "Python session"=w896) -> (w892:T2)
          }
          frame "ensure temp dir" {
            n399 = Unbundle By Name(w925) -> ("Console"=w922:refnum<vi>, "Python session"=w931:refnum<k35>, "Script path"=w930:path)
            n400 = node(w931, w930, "ensure_temp_dir" ("function name"), w929) -> (w928:errorcluster)  [unwired: 2 in, 3 out]
            n401 = property class="Str"(reference=w922) -> (reference out=w937:refnum<vi>, error out=w934:errorcluster, "Value"=w936:string)  [unwired: 1 in]
            n402 = Concatenate Strings(w936, "\n>Looking for temp directory...\n " ("function name")) -> (w935:string)
            n403 = property class="Str"(reference=w937, error in=w934, "Value"=w935) -> (reference out=w923:refnum<vi>)  [unwired: 1 out]
            n404 = case shown="Error .." w928 {
              selector: w928 -> [w952 w957]
              tunnel: w926 -> [w953 w955]
              tunnel: [w950 w956] -> w927
              tunnel: w923 -> [w939 _]
              frame No Error {
                n405 = property class="Str"(reference=w939) -> (reference out=w943:refnum<vi>, error out=w940:errorcluster, "Value"=w942:string)  [unwired: 1 in]
                n406 = Enqueue Element(queue=w953, element="adb connect", error in (no error)=w952) -> (queue out=w949:refnum<queue>, error out=w946:errorcluster)  [unwired: 1 in, 1 out]
                n407 = Concatenate Strings(w942, "Finded!" ("string")) -> (w941:string)
                n408 = Enqueue Element(queue=w949, element="clear console", error in (no error)=w946) -> (queue out=w947:refnum<queue>, error out=w945:errorcluster)  [unwired: 1 in, 1 out]
                n409 = property class="Str"(reference=w943, error in=w940, "Value"=w941) -> ()  [unwired: 2 out]
                n410 = Enqueue Element(queue=w947, element="media required", error in (no error)=w945) -> (error out=w950:errorcluster)  [unwired: 1 in, 2 out]
              }
              frame Error {
                n411 = Enqueue Element(queue=w955, element="error", error in (no error)=w957) -> (error out=w956:errorcluster)  [unwired: 1 in, 2 out]
              }
            }
          }
          frame "media required" {
            n412 = Unbundle By Name(w968) -> ("Console"=w961:refnum<vi>, "Python session"=w975:refnum<k35>, "Script path"=w974:path)
            n413 = property class="Str"(reference=w961) -> (reference out=w981:refnum<vi>, error out=w978:errorcluster, "Value"=w980:string)  [unwired: 1 in]
            n414 = Concatenate Strings(w980, ">Looking for media required...\n" ("function name")) -> (w979:string)
            n415 = property class="Str"(reference=w981, error in=w978, "Value"=w979) -> (reference out=w964:refnum<vi>, error out=w960:errorcluster)
            n416 = call "Stall Data Flow.vim"("value in"=w960, "milliseconds to wait"=u32 500) -> ("value out"=w959:errorcluster)  [unwired: 1 out]
            n417 = node(w975, w974, "get_media_required" ("function name"), w959, cluster{i32, string} {0, ""}) -> (w966:refnum<k35>, w973:errorcluster, w969:cluster{i32, string})  [unwired: 2 out]
            n418 = Unbundle(w969) -> (w962:i32, w963:string)
            n419 = Bundle By Name(cluster=w968, "Media version"=w962, "Media Url"=w963, "Python session"=w966) -> (w967:T2)
            n420 = case shown="No Error" w973 {
              selector: w973 -> [w995 w1010]
              tunnel: w971 -> [w996 w1008]
              tunnel: [w994 w1009] -> w972
              tunnel: w964 -> [w989 _]
              tunnel: w963 -> [w987 _]
              tunnel: w962 -> [w984 _]
              frame No Error {
                n421 = property class="Str"(reference=w989) -> (reference out=w993:refnum<vi>, error out=w990:errorcluster, "Value"=w992:string)  [unwired: 1 in]
                n422 = Number To Decimal String(number=w984) -> (decimal integer string=w983:string)  [unwired: 1 in]
                n423 = disable-structure shown="Enabled" {
                  disable-tunnel: w996 -> [w1000 w1002]
                  disable-tunnel: w995 -> [w999 w1003]
                  disable-tunnel: [w997 w1004] -> w994
                  frame Enabled {
                    n424 = Enqueue Element(queue=w1000, element="rm media", error in (no error)=w999) -> (error out=w997:errorcluster)  [unwired: 1 in, 2 out]
                  }
                  frame Disabled {
                    n425 = Enqueue Element(queue=w1002, element="media exist?", error in (no error)=w1003) -> (error out=w1004:errorcluster)  [unwired: 1 in, 2 out]
                  }
                }
                n426 = Concatenate Strings(w992, "Url: " ("string"), w987, "\r", "Version: #" ("string"), w983, "\r") -> (w991:string)
                n427 = property class="Str"(reference=w993, error in=w990, "Value"=w991) -> ()  [unwired: 2 out]
              }
              frame Error {
                n428 = One Button Dialog(message="------------------------------------\nFatal error opening labview script\n------------------------------------", button name ("OK")="Abort!") -> ()  [unwired: 1 out]
                n429 = Enqueue Element(queue=w1008, element="error", error in (no error)=w1010) -> (error out=w1009:errorcluster)  [unwired: 1 in, 2 out]
              }
            }
          }
          frame "media exist?" {
            n430 = Unbundle By Name(w1023) -> ("Media version"=w1018:i32)
            n431 = Number To Decimal String(number=w1018) -> (decimal integer string=w1020:string)  [unwired: 1 in]
            n432 = Concatenate Strings(w1020, ".zip" ("string")) -> (w1021:string)
            n433 = String To Path(string=w1021) -> (path=w1017:path)
            n434 = Build Path(base path=path "C:/GUIMedia", name or relative path=w1017) -> (appended path=w1016:path)
            n435 = call <vilib>:"Check if File or Folder Exists.vi"("path"=w1016) -> ("file or folder exists?"=w1015:bool)  [unwired: 8 in, 2 out]
            n436 = case shown="False" w1015 {
              tunnel: w1014 -> [w1025 w1029]
              tunnel: w1013 -> [w1027 w1031]
              tunnel: [w1024 w1028] -> w1011
              frame True {
                n437 = Enqueue Element(queue=w1025, element="rm media", error in (no error)=w1027) -> (error out=w1024:errorcluster)  [unwired: 1 in, 2 out]
              }
              frame False {
                n438 = Enqueue Element(queue=w1029, element="download", error in (no error)=w1031) -> (error out=w1028:errorcluster)  [unwired: 1 in, 2 out]
              }
            }
          }
          frame "download" {
            n439 = Unbundle By Name(w1040) -> ("Version path"=w1039:path)
            n440 = flat-sequence {
              tunnel: w1039 -> [w1044]
              tunnel: w1035 -> [w1041]
              tunnel: [w1041] -> w1034
              tunnel: w1034 -> [w1047]
              tunnel: [w1047] -> w1033
              frame #0 {
                n441 = call <vilib>:"System Exec.vi"("wait until completion? (T)"=FALSE, "working directory"=w1044, "command line"="python Update_Media.py") -> ()  [unwired: 5 in, 4 out]
              }
              frame #1 {
                n442 = One Button Dialog(message="Espere a termine el script y presione continuar", button name ("OK")="Continuar") -> ()  [unwired: 1 out]
              }
            }
            n443 = Enqueue Element(queue=w1033, element="end", error in (no error)=w1037) -> (error out=w1036:errorcluster)  [unwired: 1 in, 2 out]
          }
          frame "rm media" {
            n444 = Unbundle By Name(w1051) -> ("Console"=w1056:refnum<vi>, "Version path"=w1048:path)
            n445 = property class="Str"(reference=w1056) -> (reference out=w1057:refnum<vi>, "Value"=w1055:string)  [unwired: 1 in, 1 out]
            n446 = Concatenate Strings(w1055, "\n>rm -r -f /sdcard/media\n") -> (w1054:string)
            n447 = property class="Str"(reference=w1057, "Value"=w1054) -> (reference out=w1052:refnum<vi>)  [unwired: 1 in, 1 out]
            n448 = call <vilib>:"System Exec.vi"("run minimized? (F)"=TRUE, "working directory"=w1048, "command line"="adb shell rm -r -f /sdcard/media") -> ("error out"=w1050:errorcluster, "standard error"=w1059:string, "standard output"=w1064:string)  [unwired: 5 in, 1 out]
            n449 = property class="Str"(reference=w1052) -> (reference out=w1068:refnum<vi>, error out=w1065:errorcluster, "Value"=w1067:string)  [unwired: 1 in]
            n450 = Concatenate Strings(w1067, w1064, w1059) -> (w1066:string)
            n451 = property class="Str"(reference=w1068, error in=w1065, "Value"=w1066) -> (reference out=w1049:refnum<vi>)  [unwired: 1 out]
            n452 = case shown="No Error" w1050 {
              selector: w1050 -> [w1075 w1079]
              tunnel: w1063 -> [w1078 _]
              tunnel: [w1077 w1079] -> w1058
              tunnel: w1049 -> [w1070 _]
              frame No Error {
                n453 = property class="Str"(reference=w1070) -> (reference out=w1069:refnum<vi>, error out=w1074:errorcluster, "Value"=w1073:string)  [unwired: 1 in]
                n454 = Concatenate Strings(w1073, "Done!" ("string")) -> (w1072:string)
                n455 = property class="Str"(reference=w1069, error in=w1074, "Value"=w1072) -> ()  [unwired: 2 out]
                n456 = Enqueue Element At Opposite End(queue=w1078, element="mkdir media", error in (no error)=w1075) -> (error out=w1077:errorcluster)  [unwired: 1 in, 2 out]
              }
              frame Error {
              }
            }
          }
          frame "mkdir media" {
            n457 = Unbundle By Name(w1083) -> ("Console"=w1088:refnum<vi>, "Version path"=w1080:path)
            n458 = property class="Str"(reference=w1088) -> (reference out=w1089:refnum<vi>, "Value"=w1087:string)  [unwired: 1 in, 1 out]
            n459 = Concatenate Strings(w1087, "\n>mkdir /sdcard/media\n") -> (w1086:string)
            n460 = property class="Str"(reference=w1089, "Value"=w1086) -> (reference out=w1084:refnum<vi>)  [unwired: 1 in, 1 out]
            n461 = call <vilib>:"System Exec.vi"("run minimized? (F)"=TRUE, "working directory"=w1080, "command line"="adb shell mkdir /sdcard/media") -> ("error out"=w1082:errorcluster, "standard error"=w1091:string, "standard output"=w1096:string)  [unwired: 5 in, 1 out]
            n462 = property class="Str"(reference=w1084) -> (reference out=w1100:refnum<vi>, error out=w1097:errorcluster, "Value"=w1099:string)  [unwired: 1 in]
            n463 = Concatenate Strings(w1099, w1096, w1091) -> (w1098:string)
            n464 = property class="Str"(reference=w1100, error in=w1097, "Value"=w1098) -> (reference out=w1081:refnum<vi>)  [unwired: 1 out]
            n465 = case shown="No Error" w1082 {
              selector: w1082 -> [w1107 w1111]
              tunnel: w1095 -> [w1110 _]
              tunnel: [w1109 w1111] -> w1090
              tunnel: w1081 -> [w1102 _]
              frame No Error {
                n466 = property class="Str"(reference=w1102) -> (reference out=w1101:refnum<vi>, error out=w1106:errorcluster, "Value"=w1105:string)  [unwired: 1 in]
                n467 = Concatenate Strings(w1105, "Done!" ("string")) -> (w1104:string)
                n468 = Enqueue Element At Opposite End(queue=w1110, element="mkdir temp", error in (no error)=w1107) -> (error out=w1109:errorcluster)  [unwired: 1 in, 2 out]
                n469 = property class="Str"(reference=w1101, error in=w1106, "Value"=w1104) -> ()  [unwired: 2 out]
              }
              frame Error {
              }
            }
          }
          frame "mkdir temp" {
            n470 = Unbundle By Name(w1115) -> ("Console"=w1120:refnum<vi>, "Version path"=w1112:path)
            n471 = property class="Str"(reference=w1120) -> (reference out=w1121:refnum<vi>, "Value"=w1119:string)  [unwired: 1 in, 1 out]
            n472 = Concatenate Strings(w1119, "\n>shell mkdir /sdcard/media/temp\n") -> (w1118:string)
            n473 = property class="Str"(reference=w1121, "Value"=w1118) -> (reference out=w1116:refnum<vi>)  [unwired: 1 in, 1 out]
            n474 = call <vilib>:"System Exec.vi"("run minimized? (F)"=TRUE, "working directory"=w1112, "command line"="adb shell mkdir /sdcard/media/temp") -> ("error out"=w1114:errorcluster, "standard error"=w1123:string, "standard output"=w1128:string)  [unwired: 5 in, 1 out]
            n475 = property class="Str"(reference=w1116) -> (reference out=w1132:refnum<vi>, error out=w1129:errorcluster, "Value"=w1131:string)  [unwired: 1 in]
            n476 = Concatenate Strings(w1131, w1128, w1123) -> (w1130:string)
            n477 = property class="Str"(reference=w1132, error in=w1129, "Value"=w1130) -> (reference out=w1113:refnum<vi>)  [unwired: 1 out]
            n478 = case shown="No Error" w1114 {
              selector: w1114 -> [w1139 w1143]
              tunnel: w1127 -> [w1142 _]
              tunnel: [w1141 w1143] -> w1122
              tunnel: w1113 -> [w1134 _]
              frame No Error {
                n479 = property class="Str"(reference=w1134) -> (reference out=w1133:refnum<vi>, error out=w1138:errorcluster, "Value"=w1137:string)  [unwired: 1 in]
                n480 = Concatenate Strings(w1137, "Done!" ("string")) -> (w1136:string)
                n481 = Enqueue Element At Opposite End(queue=w1142, element="unzip", error in (no error)=w1139) -> (error out=w1141:errorcluster)  [unwired: 1 in, 2 out]
                n482 = property class="Str"(reference=w1133, error in=w1138, "Value"=w1136) -> ()  [unwired: 2 out]
              }
              frame Error {
              }
            }
          }
          frame "unzip" {
            n483 = Unbundle By Name(w1156) -> ("Media version"=w1155:i32, "My temp"=w1145:path)
            n484 = Number To Decimal String(number=w1155) -> (decimal integer string=w1159:string)  [unwired: 1 in]
            n485 = Concatenate Strings(w1159, ".zip" ("string")) -> (w1160:string)
            n486 = String To Path(string=w1160) -> (path=w1157:path)
            n487 = Build Path(base path=path "C:/GUIMedia", name or relative path=w1157) -> (appended path=w1146:path)
            n488 = call <vilib>:"Check if File or Folder Exists.vi"("path"=w1145) -> ("error out"=w1148:errorcluster, "file or folder exists?"=w1149:bool, "dup path"=w1144:path)  [unwired: 8 in]
            n489 = case shown="True" w1149 {
              tunnel: [w1163 w1169] -> _
              tunnel: [w1162 w1168] -> w1147
              tunnel: w1148 -> [w1164 w1170]
              tunnel: w1144 -> [_ w1165]
              frame False {
                n490 = Create Folder(error in=w1164) -> (created path=w1163:path, error out=w1162:errorcluster)  [unwired: 2 in, 1 out]
              }
              frame True {
                n491 = Delete(path (use dialog)=w1165, entire hierarchy (F)=TRUE, error in=w1170) -> (deleted path=w1167:path, error out=w1166:errorcluster)  [unwired: 2 in, 1 out]
                n492 = Create Folder(path (use dialog)=w1167, error in=w1166) -> (created path=w1169:path, error out=w1168:errorcluster)  [unwired: 1 in, 1 out]
              }
            }
            n493 = call <vilib>:"Unzip.vi"("error in (no error)"=w1147, "Target directory (same as Zip file if empty)"=w1145, "Zip file"=w1146) -> ()  [unwired: 6 in, 3 out]
            n494 = Enqueue Element(queue=w1152, element="send files", error in (no error)=w1153) -> (error out=w1154:errorcluster)  [unwired: 1 in, 2 out]
          }
          frame "send files" {
            w1178 = "\"" ("input 1")
            n495 = Unbundle By Name(w1183) -> ("Console"=w1187:refnum<vi>, "Version path"=w1173:path, "My temp"=w1172:path)
            n496 = property class="Str"(reference=w1187) -> (reference out=w1188:refnum<vi>, "Value"=w1186:string)  [unwired: 1 in, 1 out]
            n497 = call "Progress bar v2.vi"("TIme (s)"=130.0, "Title"="Sending media") -> ()  [unwired: 9 in, 1 out]
            n498 = Concatenate Strings(w1186, "\nSending files...\n" ("string")) -> (w1185:string)
            n499 = Path To String(path=w1172) -> (string=w1179:string)
            n500 = property class="Str"(reference=w1188, "Value"=w1185) -> (reference out=w1184:refnum<vi>)  [unwired: 1 in, 1 out]
            n501 = Concatenate Strings("adb push " ("initial string"), w1178, w1179, w1178, " /sdcard/media/" ("input 2")) -> (w1176:string)
            n502 = call <vilib>:"System Exec.vi"("run minimized? (F)"=TRUE, "working directory"=w1173, "command line"=w1176) -> ("error out"=w1182:errorcluster, "standard error"=w1190:string, "standard output"=w1194:string)  [unwired: 5 in, 1 out]
            n503 = property class="Str"(reference=w1184) -> (reference out=w1198:refnum<vi>, error out=w1195:errorcluster, "Value"=w1197:string)  [unwired: 1 in]
            n504 = Concatenate Strings(w1197, w1194, w1190) -> (w1196:string)
            n505 = property class="Str"(reference=w1198, error in=w1195, "Value"=w1196) -> ()  [unwired: 2 out]
            n506 = case shown="No Error" w1182 {
              selector: w1182 -> [w1199 w1203]
              tunnel: w1193 -> [w1202 _]
              tunnel: [w1201 w1203] -> w1189
              frame No Error {
                n507 = call <vilib>:"Close Progress Bar.vi"() -> ()  [unwired: 10 in, 2 out]
                n508 = Enqueue Element At Opposite End(queue=w1202, element="mv temp -> media", error in (no error)=w1199) -> (error out=w1201:errorcluster)  [unwired: 1 in, 2 out]
              }
              frame Error {
                n509 = call <vilib>:"Close Progress Bar.vi"() -> ()  [unwired: 10 in, 2 out]
              }
            }
          }
          frame "mv temp -> media" {
            n510 = Unbundle By Name(w1215) -> ("Console"=w1218:refnum<vi>, "Version path"=w1204:path, "Media version"=w1211:i32)
            n511 = Format Into String(format string="adb shell mv /sdcard/media/temp /sdcard/media/%d" ("command line"), w1211) -> (resulting string=w1208:string)  [unwired: 2 in, 1 out]
            n512 = property class="Str"(reference=w1218) -> (reference out=w1219:refnum<vi>, "Value"=w1217:string)  [unwired: 1 in, 1 out]
            n513 = Concatenate Strings(w1217, "\r", ">" ("string"), w1208) -> (w1216:string)
            n514 = property class="Str"(reference=w1219, "Value"=w1216) -> (reference out=w1207:refnum<vi>)  [unwired: 1 in, 1 out]
            n515 = property class="Str"(reference=w1207, "Text.Scroll Position"=u32 4294967295) -> (reference out=w1205:refnum<vi>)  [unwired: 1 in, 1 out]
            n516 = call <vilib>:"System Exec.vi"("run minimized? (F)"=TRUE, "working directory"=w1204, "command line"=w1208) -> ("error out"=w1214:errorcluster, "standard error"=w1221:string, "standard output"=w1225:string)  [unwired: 5 in, 1 out]
            n517 = property class="Str"(reference=w1205) -> (reference out=w1229:refnum<vi>, error out=w1226:errorcluster, "Value"=w1228:string)  [unwired: 1 in]
            n518 = Concatenate Strings(w1228, w1225, w1221) -> (w1227:string)
            n519 = property class="Str"(reference=w1229, error in=w1226, "Value"=w1227) -> (reference out=w1213:refnum<vi>)  [unwired: 1 out]
            n520 = case shown="No Error" w1214 {
              selector: w1214 -> [w1230 w1234]
              tunnel: w1224 -> [w1233 _]
              tunnel: [w1232 w1234] -> w1220
              tunnel: w1213 -> [_ _]
              frame No Error {
                n521 = Enqueue Element At Opposite End(queue=w1233, element="end", error in (no error)=w1230) -> (error out=w1232:errorcluster)  [unwired: 1 in, 2 out]
              }
              frame Error {
              }
            }
          }
          frame "end" {
            n522 = flat-sequence {
              frame #0 {
                n523 = One Button Dialog(message="¡Instalación terminada!") -> ()  [unwired: 1 in, 1 out]
              }
              frame #1 {
                n524 = property on="Stop button" class="Bool (strict)"("Val(Sgnl)"=TRUE ("Value (Signaling)")) -> ()  [unwired: 2 in, 2 out]
              }
            }
          }
          frame "kill loop" {
          }
          frame "legacy install media" {
            n525 = Unbundle By Name(w1251) -> ("Console"=w1247:refnum<vi>, "Python session"=w1255:refnum<k35>, "Script path"=w1254:path, "Media version"=w1242:i32)
            n526 = property class="Str"(reference=w1247) -> (reference out=w1260:refnum<vi>, error out=w1257:errorcluster, "Value"=w1259:string)  [unwired: 1 in]
            n527 = Concatenate Strings(w1259, "\n>Installing media...\n" ("function name")) -> (w1258:string)
            n528 = property class="Str"(reference=w1260, error in=w1257, "Value"=w1258) -> (reference out=w1245:refnum<vi>, error out=w1243:errorcluster)
            n529 = node(w1255, w1254, "install_media" ("function name"), w1243, w1242, w1242) -> (w1249:refnum<k35>, w1250:errorcluster)  [unwired: 2 in, 2 out]
            n530 = Close Python Session(session in=w1249, error in=w1250) -> (11:w1248:errorcluster)
            n531 = case shown="No Error" w1248 {
              selector: w1248 -> [w1261 w1271]
              tunnel: w1252 -> [w1270 w1273]
              tunnel: [w1268 w1274] -> w1253
              tunnel: w1245 -> [w1262 _]
              frame No Error {
                n532 = disable-structure shown="Disabled" {
                  frame Disabled {
                    n533 = call <vilib>:"Close Progress Bar.vi"() -> ()  [unwired: 10 in, 2 out]
                  }
                  frame Enabled {
                  }
                }
                n534 = property class="Str"(reference=w1262) -> (reference out=w1267:refnum<vi>, error out=w1266:errorcluster, "Value"=w1265:string)  [unwired: 1 in]
                n535 = Concatenate Strings(w1265, "Done!" ("string")) -> (w1264:string)
                n536 = property class="Str"(reference=w1267, error in=w1266, "Value"=w1264) -> ()  [unwired: 2 out]
                n537 = Enqueue Element(queue=w1270, element="end", error in (no error)=w1261) -> (error out=w1268:errorcluster)  [unwired: 1 in, 2 out]
              }
              frame Error {
                n538 = disable-structure shown="Disabled" {
                  frame Disabled {
                    n539 = call <vilib>:"Close Progress Bar.vi"() -> ()  [unwired: 10 in, 2 out]
                  }
                  frame Enabled {
                  }
                }
                n540 = Enqueue Element(queue=w1273, element="error", error in (no error)=w1271) -> (error out=w1274:errorcluster)  [unwired: 1 in, 2 out]
              }
            }
          }
        }
      }
      frame Error {
        n541 = Unbundle By Name(w1284) -> ("COM"=w1282:refnum<visa-resource-name>)
        n542 = Flush Queue(queue=w1285, error in (no error)=w1281) -> (queue out=w1286:refnum<queue>, error out=w1283:errorcluster)  [unwired: 1 out]
        n543 = Enqueue Element(queue=w1286, element="idle", error in (no error)=w1283) -> (error out=w1276:errorcluster)  [unwired: 1 in, 2 out]
        n544 = VISA Close(VISA resource name=w1282, error in (no error)=w1281) -> (error out=w1275:errorcluster)
        n545 = call <vilib>:"Clear Errors.vi"("error in (no error)"=w1275) -> ()  [unwired: 5 in, 2 out]
        n546 = call <vilib>:"Simple Error Handler.vi"("error in (no error)"=w1276) -> ("code out"=w1280:i32, "error out"=w1279:errorcluster)  [unwired: 4 in, 3 out]
        n547 = call <vilib>:"Clear Errors.vi"("error in (no error)"=w1279, "specific error code to clear (0: all)"=w1280) -> ("error out"=w1278:errorcluster)  [unwired: 4 in, 1 out]
        n548 = property on="Stop button" class="Bool (strict)"(error in=w1278, "Value"=TRUE ("Value (Signaling)")) -> (error out=w1277:errorcluster)  [unwired: 1 in, 1 out]
      }
    }
  }
  n549 = while {
    shift-right: [w1294] -> w45
    shift-left: w20 -> [w1296]
    tunnel: w43 -> [w1297]
    tunnel: [w1292] -> w33
    tunnel: w18 -> [w1291]
    tunnel: w1 -> [w1290]
    stop <- w1295 stop-if-true
    # "This loop is the producer loop."
    # "Event handler"
    n550 = event shown="[4] \"Stop button\": Value Change" {
      selector: w1290 -> [_ _ _ _ _ _ _]
      dyn-events: [_ _ _ _ _ _ _] -> w1292
      timeout: _ -> [_ _ _ _ _ _ _]
      tunnel: w1297 -> [w1301 w1314 w1325 w1337 w1342 w1352 _]
      tunnel: w1296 -> [w1300 w1313 w1326 w1338 w1343 w1349 w1355]
      tunnel: [w1299 w1312 w1323 w1336 w1345 w1348 w1354] -> w1294
      tunnel: [_ _ _ _ _ _ TRUE] -> w1293
      tunnel: w1291 -> [_ _ _ w1339 w1341 _ w1356]
      event "Settings button": Value Change {
        n551 = event-data() -> ("NewVal"=w1298:bool)  [unwired: 1 in]
        n552 = case shown="False" w1298 {
          tunnel: w1301 -> [w1304 w1310]
          tunnel: w1300 -> [w1306 w1309]
          tunnel: [w1303 w1308] -> w1299
          frame False {
            n553 = Enqueue Element(queue=w1304, element="close settings", error in (no error)=w1306) -> (error out=w1303:errorcluster)  [unwired: 1 in, 2 out]
            n554 = property on="Paths" class="Bool (strict)"("Val(Sgnl)"=FALSE ("Value (Signaling)")) -> ()  [unwired: 2 in, 2 out]
          }
          frame True {
            n555 = Enqueue Element(queue=w1310, element="open settings", error in (no error)=w1309) -> (error out=w1308:errorcluster)  [unwired: 1 in, 2 out]
          }
        }
      }
      event "Paths": Value Change {
        n556 = event-data() -> ("NewVal"=w1311:bool)  [unwired: 1 in]
        n557 = case shown="True" w1311 {
          tunnel: w1314 -> [w1315 w1322]
          tunnel: w1313 -> [w1317 w1321]
          tunnel: [w1318 w1320] -> w1312
          frame False {
            n558 = Enqueue Element(queue=w1315, element="close paths", error in (no error)=w1317) -> (error out=w1318:errorcluster)  [unwired: 1 in, 2 out]
          }
          frame True {
            n559 = Enqueue Element(queue=w1322, element="open paths", error in (no error)=w1321) -> (error out=w1320:errorcluster)  [unwired: 1 in, 2 out]
          }
        }
      }
      event "Save button": Value Change {
        n560 = event-data() -> ("NewVal"=w1324:bool)  [unwired: 1 in, 2 out]
        n561 = case shown="True" w1324 {
          tunnel: w1325 -> [_ w1331]
          tunnel: w1326 -> [w1327 w1330]
          tunnel: [w1327 w1329] -> w1323
          frame False {
          }
          frame True {
            n562 = Enqueue Element(queue=w1331, element="save config", error in (no error)=w1330) -> (error out=w1329:errorcluster)  [unwired: 1 in, 2 out]
          }
        }
      }
      event "Run button": Value Change {
        n563 = event-data() -> ()  [unwired: 1 in, 6 out]
        n564 = Enqueue Element(queue=w1337, element="running") -> (error out=w1334:errorcluster)  [unwired: 2 in, 2 out]
        n565 = Enqueue Element(queue=w1339, element="validate config", error in (no error)=w1338) -> (error out=w1335:errorcluster)  [unwired: 1 in, 2 out]
        n566 = Merge Errors(w1334, w1335) -> (w1336:errorcluster)
      }
      event "Stop button": Value Change {
        n567 = event-data() -> ()  [unwired: 1 in, 6 out]
        n568 = Enqueue Element At Opposite End(queue=w1342, element="idle", error in (no error)=w1343) -> (error out=w1347:errorcluster)  [unwired: 1 in, 2 out]
        n569 = Enqueue Element At Opposite End(queue=w1341, element="idle", error in (no error)=w1343) -> (error out=w1340:errorcluster)  [unwired: 1 in, 2 out]
        n570 = Merge Errors(w1347, w1340) -> (w1345:errorcluster)
      }
      event Panel Close? {
        n571 = event-data() -> ()  [unwired: 1 in, 3 out]
        n572 = Enqueue Element At Opposite End(queue=w1352, element="confirm quit", error in (no error)=w1349) -> (error out=w1348:errorcluster)  [unwired: 1 in, 2 out]
        n573 = event-data("Discard?"=TRUE) -> ()  [unwired: 1 in, 1 out]
      }
      event User Event {
        n574 = event-data() -> ()  [unwired: 1 in, 3 out]
        n575 = Enqueue Element At Opposite End(queue=w1356, element="kill loop", error in (no error)=w1355) -> (error out=w1354:errorcluster)  [unwired: 1 in, 2 out]
      }
    }
    n576 = Or(x=w1294, y=w1293) -> (x .or. y?=w1295:bool)
  }
  n577 = control-ref of="Paths"() -> (w8:refnum<vi>)
  n578 = Bundle("secondary color"=w5, "secondary color"=w5) -> (w4:T12)  [unwired: 1 in]
  n579 = call "button painter (SubVI).vi"("Off state"=w4, "On state"=w7, "Button ref in"=w8) -> ()  [unwired: 9 in]
  n580 = while {
    tunnel: w43 -> [w1365]
    shift-right: [w1360] -> _
    shift-left: w41 -> [w1361]
    tunnel: w35 -> [w1358]
    stop <- w1363 stop-if-true
    # "This loop is a consumer loop."
    # "UI consummer"
    n581 = Dequeue Element(queue=w1365) -> (queue out=w1359:refnum<queue>, element=w1362:string, error out=w1364:errorcluster)  [unwired: 2 in, 1 out]
    n582 = case shown="No Error" w1364 {
      tunnel: [_ TRUE] -> w1363
      tunnel: w1362 -> [w1370 _]
      tunnel: w1361 -> [w1369 _]
      tunnel: [w1368 _] -> w1360
      tunnel: w1359 -> [w1367 _]
      tunnel: w1358 -> [w1366 _]
      frame No Error {
        # "Process the data here."
        n583 = case shown="\"idle\"" w1370 {
          tunnel: w1369 -> [w1381 w1393 w1397 w1405 w1422 w1429 w1435 w1446 w1453 w1460 w1467]
          tunnel: [w1380 w1393 w1397 w1405 w1422 w1429 w1435 w1446 w1453 w1460 w1467] -> w1368
          tunnel: w1367 -> [w1378 _ _ _ _ _ _ _ _ w1457 _]
          tunnel: w1366 -> [_ _ _ _ _ _ _ _ _ _ w1466]
          frame "init", Default {
            n584 = Enqueue Element(queue=w1378, element="read config") -> (queue out=w1374:refnum<queue>, error out=w1376:errorcluster)  [unwired: 2 in, 1 out]
            n585 = Enqueue Element(queue=w1374, element="idle", error in (no error)=w1376) -> ()  [unwired: 1 in, 3 out]
            n586 = control-ref of="footer splitter"() -> (w1379:refnum<vi>)
            n587 = control-ref of="Serial communication\n settings"() -> (w1371:refnum<vi>)
            n588 = control-ref of="Path: Android OS"() -> (w1373:refnum<vi>)
            n589 = control-ref of="Path: 4.9.12.XXXX"() -> (w1372:refnum<vi>)
            n590 = control-ref of="settings splitter"() -> (w1382:refnum<vi>)
            n591 = Bundle By Name(cluster=w1381, "settings splitter"=w1382, "footer splitter"=w1379, "Serial communication\n settings"=w1371, "Path: Android OS"=w1373, "Path: 4.9.12.XXXX"=w1372) -> (w1380:T4)
          }
          frame "idle" {
            n592 = property on="Save button" class="Bool (strict)"("DisabledEnum"=T3."Enabled" ("Disabled"), "Value"=FALSE ("Save button")) -> ()  [unwired: 2 in, 2 out]
            n593 = property on="Settings button" class="Bool (strict)"("DisabledEnum"=T3."Enabled" ("Disabled"), "Val(Sgnl)"=FALSE ("Settings")) -> ()  [unwired: 2 in, 2 out]
            n594 = property on="Run button" class="Bool (strict)"("DisabledEnum"=T3."Enabled" ("Disabled"), "Value"=FALSE ("Save button")) -> ()  [unwired: 2 in, 2 out]
            n595 = property on="Stop button" class="Bool (strict)"("DisabledEnum"=T3."Disabled" ("Disabled"), "Value"=FALSE ("Save button")) -> ()  [unwired: 2 in, 2 out]
            n596 = property on="Paths" class="Bool (strict)"("DisabledEnum"=T3."Enabled" ("Disabled"), "Val(Sgnl)"=FALSE ("Paths")) -> ()  [unwired: 2 in, 2 out]
          }
          frame "running" {
            n597 = property on="Run button" class="Bool (strict)"("DisabledEnum"=T3."Disabled" ("Disabled")) -> ()  [unwired: 2 in, 2 out]
            n598 = property on="Stop button" class="Bool (strict)"("Value"=TRUE ("Stop button"), "DisabledEnum"=T3."Enabled" ("Disabled")) -> ()  [unwired: 2 in, 2 out]
          }
          frame "read config" {
            n599 = Unbundle By Name(w1405) -> ("Path: Android OS"=w1400:refnum<vi>, "Path: 4.9.12.XXXX"=w1403:refnum<vi>, "Serial communication\n settings"=w1404:refnum<vi>)
            n600 = call "settings handler.vi"("Operation"=enum16{"Open", "Write", "Read", "Close"}."Open") -> ("Error Out"=w1408:errorcluster)  [unwired: 8 in, 2 out]
            n601 = call "settings handler.vi"("Operation"=enum16{"Open", "Write", "Read", "Close"}."Read", "error in (no error)"=w1408) -> ("Paths read"=w1402:T10, "Read"=w1398:T1)  [unwired: 7 in, 1 out]
            n602 = property class="Clust (strict)"(reference=w1404, "Value"=w1398) -> ()  [unwired: 1 in, 2 out]
            n603 = Unbundle By Name(w1402) -> ("Version"=w1401:path, "Android"=w1399:path)
            n604 = property class="Path"(reference=w1403, "Value"=w1401) -> ()  [unwired: 1 in, 2 out]
            n605 = property class="Path"(reference=w1400, "Value"=w1399) -> ()  [unwired: 1 in, 2 out]
          }
          frame "save config" {
            n606 = Unbundle By Name(w1422) -> ("Serial communication\n settings"=w1421:refnum<vi>, "Path: Android OS"=w1418:refnum<vi>, "Path: 4.9.12.XXXX"=w1417:refnum<vi>)
            n607 = property class="Path"(reference=w1417) -> ("Value"=w1415:path)  [unwired: 1 in, 2 out]
            n608 = property on="Save button" class="Bool (strict)"("Value"=FALSE ("Save button")) -> ()  [unwired: 2 in, 2 out]
            n609 = property class="Clust (strict)"(reference=w1421) -> ("Value"=w1413:T1)  [unwired: 1 in, 2 out]
            n610 = property class="Path"(reference=w1418) -> ("Value"=w1416:path)  [unwired: 1 in, 2 out]
            n611 = Bundle("Value"=w1416, "Value"=w1415, path "", path "", path "") -> (w1414:T13)  [unwired: 1 in]
            n612 = call "settings handler.vi"("Operation"=enum16{"Open", "Write", "Read", "Close"}."Write", "Paths write"=w1414, "Write"=w1413) -> ("Error Out"=w1412:errorcluster)  [unwired: 6 in, 2 out]
            n613 = case shown="No Error" w1412 {
              selector: w1412 -> [w1425 _]
              frame No Error {
                n614 = call "settings handler.vi"("Operation"=enum16{"Open", "Write", "Read", "Close"}."Close", "error in (no error)"=w1425) -> ("Error Out"=w1423:errorcluster)  [unwired: 7 in, 2 out]
                n615 = call "settings handler.vi"("Operation"=enum16{"Open", "Write", "Read", "Close"}."Open", "error in (no error)"=w1423) -> ()  [unwired: 7 in, 3 out]
                n616 = One Button Dialog(message="¡Se ha guardado con éxito!") -> ()  [unwired: 1 in, 1 out]
              }
              frame Error {
                n617 = One Button Dialog(message="¡Se ha producido un error al guardar!") -> ()  [unwired: 1 in, 1 out]
              }
            }
          }
          frame "open settings" {
            n618 = Unbundle By Name(w1429) -> ("settings splitter"=w1431:refnum<vi>, "footer splitter"=w1430:refnum<vi>)
            n619 = property class="Splitter"(reference=w1430) -> ("Width"=w1434:u32)  [unwired: 1 in, 2 out]
            n620 = Subtract(x=w1434, y=u32 240) -> (x-y=w1433:u32)
            n621 = property class="Splitter"(reference=w1431, "Position"=w1433) -> ()  [unwired: 1 in, 2 out]
          }
          frame "close settings" {
            n622 = Unbundle By Name(w1435) -> ("settings splitter"=w1437:refnum<vi>, "footer splitter"=w1436:refnum<vi>)
            n623 = property class="Splitter"(reference=w1436) -> ("Width"=w1440:u32)  [unwired: 1 in, 2 out]
            n624 = Subtract(x=w1440, y=u32 6) -> (x-y=w1439:u32)
            n625 = property class="Splitter"(reference=w1437, "Position"=w1439) -> ()  [unwired: 1 in, 2 out]
          }
          frame "open paths" {
            n626 = control-ref of="This VI"() -> (w1445:refnum<vi>)
            n627 = Unbundle By Name(w1446) -> ("footer splitter"=w1447:refnum<vi>)
            n628 = property class="VI"(reference=w1445) -> ("Panel"=w1444:refnum<vi>)  [unwired: 1 in, 2 out]
            n629 = property class="Pnl"(reference=w1444) -> ("Height"=w1443:u32)  [unwired: 1 in, 2 out]
            n630 = Subtract(x=w1443, y=u32 125) -> (x-y=w1441:u32)
            n631 = property class="Splitter"(reference=w1447, "Position"=w1441) -> ()  [unwired: 1 in, 2 out]
          }
          frame "close paths" {
            n632 = control-ref of="This VI"() -> (w1452:refnum<vi>)
            n633 = Unbundle By Name(w1453) -> ("footer splitter"=w1454:refnum<vi>)
            n634 = property class="VI"(reference=w1452) -> ("Panel"=w1451:refnum<vi>)  [unwired: 1 in, 2 out]
            n635 = property class="Pnl"(reference=w1451) -> ("Height"=w1450:u32)  [unwired: 1 in, 2 out]
            n636 = Subtract(x=w1450, y=u32 28) -> (x-y=w1449:u32)
            n637 = property class="Splitter"(reference=w1454, "Position"=w1449) -> ()  [unwired: 1 in, 2 out]
          }
          frame "confirm quit" {
            n638 = Two Button Dialog(message="¿Seguro que quiere cerrar\nla aplicación?", 1:"Cancelar" ("F button name (\"Cancel\")"), 2:"Si" ("T button name (\"OK\")")) -> (T button?=w1459:bool)
            n639 = case shown="True" w1459 {
              tunnel: w1457 -> [_ w1462]
              frame False {
              }
              frame True {
                n640 = Enqueue Element At Opposite End(queue=w1462, element="exit" ("Message")) -> ()  [unwired: 2 in, 3 out]
              }
            }
          }
          frame "exit" {
            n641 = call "settings handler.vi"("Operation"=enum16{"Open", "Write", "Read", "Close"}."Close") -> ("Error Out"=w1464:errorcluster)  [unwired: 8 in, 2 out]
            n642 = Generate User Event(user event=w1466, event data cluster="stop app" ("event data"), error in=w1464) -> ()  [unwired: 1 in, 2 out]
          }
        }
      }
      frame Error {
        # "Return true in any case that should stop the loop."
      }
    }
  }
  n643 = Release Queue(queue=w43, error in (no error)=w45) -> (error out=w34:errorcluster)  [unwired: 1 in, 2 out]
  n644 = Unregister For Events(event registration refnum=w33, error in=w34) -> (error out=w19:errorcluster)
  n645 = Release Queue(queue=w18, error in (no error)=w19) -> ()  [unwired: 1 in, 3 out]
